vi "PH_DataViewer.Read Data from Disk.vi"(5 "error in":errorcluster) -> (8 "Version":u8, 9 "new file path":path, 10 "Data Vers 1":T31 {"BNC555s"."BNC555 ConfigData"."Configuration"."System"."To Gate Polarity" items=["Low", "High"]; "BNC555s"."BNC555 ConfigData"."Configuration"."System"."To Trigger Edge" items=["Rising", "Falling"]; "BNC555s"."BNC555 ConfigData"."Configuration"."System"."To Trigger Threshold" min=0.2 max=12 step=0.01 format="%.2f"; "BNC555s"."BNC555 ConfigData"."Configuration"."System"."To DCycle Off Count" min=1 max=50000 step=1; "BNC555s"."BNC555 ConfigData"."Configuration"."System"."To DCycle On Count" min=1 max=50000 step=1; "BNC555s"."BNC555 ConfigData"."Configuration"."System"."To Burst Count" min=1 max=50000 step=1; "BNC555s"."BNC555 ConfigData"."Configuration"."System"."To Trigger Mode" items=["Disabled", "Trigger", "Gate"]; "BNC555s"."BNC555 ConfigData"."Configuration"."System"."To Mode" items=["Normal", "Single", "Burst", "DCycle"]; "BNC555s"."BNC555 ConfigData"."Configuration"."System"."To Period" min=1e-06 max=20.0 step=1e-07 format="%.7f"; "BNC555s"."BNC555 ConfigData"."Configuration"."System"."To State" items=["Disabled", "Enable"]; "BNC555s"."BNC555 ConfigData"."Channel Array"."Channel Setup"."Ch Divide By Count" min=1 max=50000 step=1; "BNC555s"."BNC555 ConfigData"."Channel Array"."Channel Setup"."Ch Burst Count" min=1 max=50000 step=1; "BNC555s"."BNC555 ConfigData"."Channel Array"."Channel Setup"."Ch Mode" items=["Normal", "Single", "Burst", "Divide by"]; "BNC555s"."BNC555 ConfigData"."Channel Array"."Channel Setup"."Ch Gate" items=["Disabled", "Enabled"]; "BNC555s"."BNC555 ConfigData"."Channel Array"."Channel Setup"."Ch Gate Polarity" items=["Normal", "Complement"]; "BNC555s"."BNC555 ConfigData"."Channel Array"."Channel Setup"."Ch Polarity" items=["Normal", "Complement"]; "BNC555s"."BNC555 ConfigData"."Channel Array"."Channel Setup"."Ch Amplitude" min=1.99 max=12 step=0.01 format="%.2f"; "BNC555s"."BNC555 ConfigData"."Channel Array"."Channel Setup"."Ch Output" items=["TTL", "Adjustable"]; "BNC555s"."BNC555 ConfigData"."Channel Array"."Channel Setup"."Ch Delay" min=0.0 max=20.0 step=1e-09 format="%.9f"; "BNC555s"."BNC555 ConfigData"."Channel Array"."Channel Setup"."Ch Width" min=4e-09 max=20.0 step=1e-09 format="%.9f"; "BNC555s"."BNC555 ConfigData"."Channel Array"."Channel Setup"."Ch State" items=["Disabled", "Enable"]; "PP PUs"."State" items=["no info", "off/false/out", "on/true/in", "Failure", "Alarm", "Status 1", "Status 2", "Status 3"]; "Chillers"."State Niveau" items=["no info", "off/false", "on/true", "Failure", "Alarm"]; "Chillers"."State Temperature" items=["no info", "off/false", "on/true", "Failure", "Alarm"]; "Chillers"."State Conductivity" items=["no info", "off/false", "on/true", "Failure", "Alarm"]; "Chillers"."State Flow" items=["no info", "off/false", "on/true", "Failure", "Alarm"]; "Mercury Monitors"."Concentration [mg/m³]" format="%#_9g"; "Mercury Monitors"."State Alarm" items=["no info", "off/false", "on/true", "Failure", "Alarm"]; "Mercury Monitors"."State On/Off" items=["no info", "off/false", "on/true", "Failure", "Alarm"]; "Img Operators"."Energy"."State" items=["no info", "off/false", "on/true", "Failure", "Alarm"]; "Img Operators"."Cam Settings"."Serial Number" format="%#_12g"; "Img Operators"."Calibration"."Calibration data - Version 1"."Cam Settings"."Serial Number" format="%#_12g"; "Img Operators"."Calibration"."Status" items=["no info", "off/false", "on/true", "Failure", "Alarm"]; "Cams"."Cam Settings"."Serial Number" format="%#_12g"; "Powermeters"."Device State" items=["no info", "off/false", "on/true", "Failure", "Alarm"]; "Calorimeters"."PH Calorimeter Device Config"."Channel Gain" items=["Range: +/- 10 V", "Range: +/- 2.5 V ", "Range: +/- 1 V", "Range: +/- 0.25 V", "Range: +/- 0.1 V", "Range: +/- 0.025 V"]; "Calorimeters"."PH Calorimeter Device Config"."Channel" items=["Channel 1", "Channel 2", "Channel 3", "Channel 4", "Channel 5", "Channel 6", "Channel 7", "Channel 8", "Channel 9", "Channel 10", "Channel 11", "Channel 12", "Channel 13", "Channel 14", "Channel 15", "Channel 16"]; "Black Boxes"."Status" items=["no info", "off/false", "on/true", "Failure", "Alarm", "Status 1", "Status 2", "Status 3"]}, 12 "Data Vers 2":T32 {"SRDG535s"."Trigger Settings"."Burst Period" min=4 max=32766; "SRDG535s"."Trigger Settings"."Internal/Burst Rate (Hz)" min=0.001 max=1000000.0 format="%.3f"; "SRDG535s"."Trigger Settings"."external level (V)" min=-2.56 max=2.56 format="%.2f"; "SRDG535s"."Trigger Settings"."burst count" min=2 max=32766; "SRDG535s"."Trigger Settings"."trigger" scale=0.0..4.0; "SRDG535s"."Output Settings"."CH CD"."Mode" items=["TTL", "NIM", "ECL", "VAR"]; "SRDG535s"."Output Settings"."CH CD"."Offset (V)" min=-3.0 max=4.0 format="%.2f"; "SRDG535s"."Output Settings"."CH CD"."Amplitude (V)" min=-3.0 max=4.0 format="%.2f"; "SRDG535s"."Output Settings"."CH D"."Mode" items=["TTL", "NIM", "ECL", "VAR"]; "SRDG535s"."Output Settings"."CH D"."Offset (V)" min=-3.0 max=4.0 format="%.2f"; "SRDG535s"."Output Settings"."CH D"."Amplitude (V)" min=-3.0 max=4.0 format="%.2f"; "SRDG535s"."Output Settings"."CH C"."Mode" items=["TTL", "NIM", "ECL", "VAR"]; "SRDG535s"."Output Settings"."CH C"."Offset (V)" min=-3.0 max=4.0 format="%.2f"; "SRDG535s"."Output Settings"."CH C"."Amplitude (V)" min=-3.0 max=4.0 format="%.2f"; "SRDG535s"."Output Settings"."CH AB"."Mode" items=["TTL", "NIM", "ECL", "VAR"]; "SRDG535s"."Output Settings"."CH AB"."Offset (V)" min=-3.0 max=4.0 format="%.2f"; "SRDG535s"."Output Settings"."CH AB"."Amplitude (V)" min=-3.0 max=4.0 format="%.2f"; "SRDG535s"."Output Settings"."CH B"."Mode" items=["TTL", "NIM", "ECL", "VAR"]; "SRDG535s"."Output Settings"."CH B"."Offset (V)" min=-3.0 max=4.0 format="%.2f"; "SRDG535s"."Output Settings"."CH B"."Amplitude (V)" min=-3.0 max=4.0 format="%.2f"; "SRDG535s"."Output Settings"."CH A"."Mode" items=["TTL", "NIM", "ECL", "VAR"]; "SRDG535s"."Output Settings"."CH A"."Offset (V)" min=-3.0 max=4.0 format="%.2f"; "SRDG535s"."Output Settings"."CH A"."Amplitude (V)" min=-3.0 max=4.0 format="%.2f"; "SRDG535s"."Output Settings"."CH T0"."Mode" items=["TTL", "NIM", "ECL", "VAR"]; "SRDG535s"."Output Settings"."CH T0"."Offset (V)" min=-3.0 max=4.0 format="%.2f"; "SRDG535s"."Output Settings"."CH T0"."Amplitude (V)" min=-3.0 max=4.0 format="%.2f"; "SRDG535s"."Delay Settings"."CH D"."Delay (s)" format="%#_13g"; "SRDG535s"."Delay Settings"."CH D"."rel to" scale=0.0..3.0; "SRDG535s"."Delay Settings"."CH C"."Delay (s)" format="%#_13g"; "SRDG535s"."Delay Settings"."CH C"."rel to" scale=0.0..3.0; "SRDG535s"."Delay Settings"."CH B"."Delay (s)" format="%#_13g"; "SRDG535s"."Delay Settings"."CH B"."rel to" scale=0.0..3.0; "SRDG535s"."Delay Settings"."CH A"."Delay (s)" format="%#_13g"; "SRDG535s"."Delay Settings"."CH A"."rel to" scale=0.0..3.0; "BNC555s"."BNC555 ConfigData"."Configuration"."System"."To Gate Polarity" items=["Low", "High"]; "BNC555s"."BNC555 ConfigData"."Configuration"."System"."To Trigger Edge" items=["Rising", "Falling"]; "BNC555s"."BNC555 ConfigData"."Configuration"."System"."To Trigger Threshold" min=0.2 max=12 step=0.01 format="%.2f"; "BNC555s"."BNC555 ConfigData"."Configuration"."System"."To DCycle Off Count" min=1 max=50000 step=1; "BNC555s"."BNC555 ConfigData"."Configuration"."System"."To DCycle On Count" min=1 max=50000 step=1; "BNC555s"."BNC555 ConfigData"."Configuration"."System"."To Burst Count" min=1 max=50000 step=1; "BNC555s"."BNC555 ConfigData"."Configuration"."System"."To Trigger Mode" items=["Disabled", "Trigger", "Gate"]; "BNC555s"."BNC555 ConfigData"."Configuration"."System"."To Mode" items=["Normal", "Single", "Burst", "DCycle"]; "BNC555s"."BNC555 ConfigData"."Configuration"."System"."To Period" min=1e-06 max=20.0 step=1e-07 format="%.7f"; "BNC555s"."BNC555 ConfigData"."Configuration"."System"."To State" items=["Disabled", "Enable"]; "BNC555s"."BNC555 ConfigData"."Channel Array"."Channel Setup"."Ch Divide By Count" min=1 max=50000 step=1; "BNC555s"."BNC555 ConfigData"."Channel Array"."Channel Setup"."Ch Burst Count" min=1 max=50000 step=1; "BNC555s"."BNC555 ConfigData"."Channel Array"."Channel Setup"."Ch Mode" items=["Normal", "Single", "Burst", "Divide by"]; "BNC555s"."BNC555 ConfigData"."Channel Array"."Channel Setup"."Ch Gate" items=["Disabled", "Enabled"]; "BNC555s"."BNC555 ConfigData"."Channel Array"."Channel Setup"."Ch Gate Polarity" items=["Normal", "Complement"]; "BNC555s"."BNC555 ConfigData"."Channel Array"."Channel Setup"."Ch Polarity" items=["Normal", "Complement"]; "BNC555s"."BNC555 ConfigData"."Channel Array"."Channel Setup"."Ch Amplitude" min=1.99 max=12 step=0.01 format="%.2f"; "BNC555s"."BNC555 ConfigData"."Channel Array"."Channel Setup"."Ch Output" items=["TTL", "Adjustable"]; "BNC555s"."BNC555 ConfigData"."Channel Array"."Channel Setup"."Ch Delay" min=0.0 max=20.0 step=1e-09 format="%.9f"; "BNC555s"."BNC555 ConfigData"."Channel Array"."Channel Setup"."Ch Width" min=4e-09 max=20.0 step=1e-09 format="%.9f"; "BNC555s"."BNC555 ConfigData"."Channel Array"."Channel Setup"."Ch State" items=["Disabled", "Enable"]; "PP PUs"."State" items=["no info", "off/false/out", "on/true/in", "Failure", "Alarm", "Status 1", "Status 2", "Status 3"]; "Chillers"."State Niveau" items=["no info", "off/false", "on/true", "Failure", "Alarm"]; "Chillers"."State Temperature" items=["no info", "off/false", "on/true", "Failure", "Alarm"]; "Chillers"."State Conductivity" items=["no info", "off/false", "on/true", "Failure", "Alarm"]; "Chillers"."State Flow" items=["no info", "off/false", "on/true", "Failure", "Alarm"]; "Mercury Monitors"."Concentration [mg/m³]" format="%#_9g"; "Mercury Monitors"."State Alarm" items=["no info", "off/false", "on/true", "Failure", "Alarm"]; "Mercury Monitors"."State On/Off" items=["no info", "off/false", "on/true", "Failure", "Alarm"]; "Img Operators"."Energy"."State" items=["no info", "off/false", "on/true", "Failure", "Alarm"]; "Img Operators"."Cam Settings"."Serial Number" format="%#_12g"; "Img Operators"."Calibration"."Calibration data - Version 1"."Cam Settings"."Serial Number" format="%#_12g"; "Img Operators"."Calibration"."Status" items=["no info", "off/false", "on/true", "Failure", "Alarm"]; "Cams"."Cam Settings"."Serial Number" format="%#_12g"; "Powermeters"."Device State" items=["no info", "off/false", "on/true", "Failure", "Alarm"]; "Calorimeters"."PH Calorimeter Device Config"."Channel Gain" items=["Range: +/- 10 V", "Range: +/- 2.5 V ", "Range: +/- 1 V", "Range: +/- 0.25 V", "Range: +/- 0.1 V", "Range: +/- 0.025 V"]; "Calorimeters"."PH Calorimeter Device Config"."Channel" items=["Channel 1", "Channel 2", "Channel 3", "Channel 4", "Channel 5", "Channel 6", "Channel 7", "Channel 8", "Channel 9", "Channel 10", "Channel 11", "Channel 12", "Channel 13", "Channel 14", "Channel 15", "Channel 16"]; "Black Boxes"."Status" items=["no info", "off/false", "on/true", "Failure", "Alarm", "Status 1", "Status 2", "Status 3"]}, 14 "Data Vers 3":T33 {"Backreflection Meas"."Waveform Data"."Initial X" format="%.2e"; "SRDG535s"."Trigger Settings"."Burst Period" min=4 max=32766; "SRDG535s"."Trigger Settings"."Internal/Burst Rate (Hz)" min=0.001 max=1000000.0 format="%.3f"; "SRDG535s"."Trigger Settings"."external level (V)" min=-2.56 max=2.56 format="%.2f"; "SRDG535s"."Trigger Settings"."burst count" min=2 max=32766; "SRDG535s"."Trigger Settings"."trigger" scale=0.0..4.0; "SRDG535s"."Output Settings"."CH CD"."Mode" items=["TTL", "NIM", "ECL", "VAR"]; "SRDG535s"."Output Settings"."CH CD"."Offset (V)" min=-3.0 max=4.0 format="%.2f"; "SRDG535s"."Output Settings"."CH CD"."Amplitude (V)" min=-3.0 max=4.0 format="%.2f"; "SRDG535s"."Output Settings"."CH D"."Mode" items=["TTL", "NIM", "ECL", "VAR"]; "SRDG535s"."Output Settings"."CH D"."Offset (V)" min=-3.0 max=4.0 format="%.2f"; "SRDG535s"."Output Settings"."CH D"."Amplitude (V)" min=-3.0 max=4.0 format="%.2f"; "SRDG535s"."Output Settings"."CH C"."Mode" items=["TTL", "NIM", "ECL", "VAR"]; "SRDG535s"."Output Settings"."CH C"."Offset (V)" min=-3.0 max=4.0 format="%.2f"; "SRDG535s"."Output Settings"."CH C"."Amplitude (V)" min=-3.0 max=4.0 format="%.2f"; "SRDG535s"."Output Settings"."CH AB"."Mode" items=["TTL", "NIM", "ECL", "VAR"]; "SRDG535s"."Output Settings"."CH AB"."Offset (V)" min=-3.0 max=4.0 format="%.2f"; "SRDG535s"."Output Settings"."CH AB"."Amplitude (V)" min=-3.0 max=4.0 format="%.2f"; "SRDG535s"."Output Settings"."CH B"."Mode" items=["TTL", "NIM", "ECL", "VAR"]; "SRDG535s"."Output Settings"."CH B"."Offset (V)" min=-3.0 max=4.0 format="%.2f"; "SRDG535s"."Output Settings"."CH B"."Amplitude (V)" min=-3.0 max=4.0 format="%.2f"; "SRDG535s"."Output Settings"."CH A"."Mode" items=["TTL", "NIM", "ECL", "VAR"]; "SRDG535s"."Output Settings"."CH A"."Offset (V)" min=-3.0 max=4.0 format="%.2f"; "SRDG535s"."Output Settings"."CH A"."Amplitude (V)" min=-3.0 max=4.0 format="%.2f"; "SRDG535s"."Output Settings"."CH T0"."Mode" items=["TTL", "NIM", "ECL", "VAR"]; "SRDG535s"."Output Settings"."CH T0"."Offset (V)" min=-3.0 max=4.0 format="%.2f"; "SRDG535s"."Output Settings"."CH T0"."Amplitude (V)" min=-3.0 max=4.0 format="%.2f"; "SRDG535s"."Delay Settings"."CH D"."Delay (s)" format="%#_13g"; "SRDG535s"."Delay Settings"."CH D"."rel to" scale=0.0..3.0; "SRDG535s"."Delay Settings"."CH C"."Delay (s)" format="%#_13g"; "SRDG535s"."Delay Settings"."CH C"."rel to" scale=0.0..3.0; "SRDG535s"."Delay Settings"."CH B"."Delay (s)" format="%#_13g"; "SRDG535s"."Delay Settings"."CH B"."rel to" scale=0.0..3.0; "SRDG535s"."Delay Settings"."CH A"."Delay (s)" format="%#_13g"; "SRDG535s"."Delay Settings"."CH A"."rel to" scale=0.0..3.0; "BNC555s"."BNC555 ConfigData"."Configuration"."System"."To Gate Polarity" items=["Low", "High"]; "BNC555s"."BNC555 ConfigData"."Configuration"."System"."To Trigger Edge" items=["Rising", "Falling"]; "BNC555s"."BNC555 ConfigData"."Configuration"."System"."To Trigger Threshold" min=0.2 max=12 step=0.01 format="%.2f"; "BNC555s"."BNC555 ConfigData"."Configuration"."System"."To DCycle Off Count" min=1 max=50000 step=1; "BNC555s"."BNC555 ConfigData"."Configuration"."System"."To DCycle On Count" min=1 max=50000 step=1; "BNC555s"."BNC555 ConfigData"."Configuration"."System"."To Burst Count" min=1 max=50000 step=1; "BNC555s"."BNC555 ConfigData"."Configuration"."System"."To Trigger Mode" items=["Disabled", "Trigger", "Gate"]; "BNC555s"."BNC555 ConfigData"."Configuration"."System"."To Mode" items=["Normal", "Single", "Burst", "DCycle"]; "BNC555s"."BNC555 ConfigData"."Configuration"."System"."To Period" min=1e-06 max=20.0 step=1e-07 format="%.7f"; "BNC555s"."BNC555 ConfigData"."Configuration"."System"."To State" items=["Disabled", "Enable"]; "BNC555s"."BNC555 ConfigData"."Channel Array"."Channel Setup"."Ch Divide By Count" min=1 max=50000 step=1; "BNC555s"."BNC555 ConfigData"."Channel Array"."Channel Setup"."Ch Burst Count" min=1 max=50000 step=1; "BNC555s"."BNC555 ConfigData"."Channel Array"."Channel Setup"."Ch Mode" items=["Normal", "Single", "Burst", "Divide by"]; "BNC555s"."BNC555 ConfigData"."Channel Array"."Channel Setup"."Ch Gate" items=["Disabled", "Enabled"]; "BNC555s"."BNC555 ConfigData"."Channel Array"."Channel Setup"."Ch Gate Polarity" items=["Normal", "Complement"]; "BNC555s"."BNC555 ConfigData"."Channel Array"."Channel Setup"."Ch Polarity" items=["Normal", "Complement"]; "BNC555s"."BNC555 ConfigData"."Channel Array"."Channel Setup"."Ch Amplitude" min=1.99 max=12 step=0.01 format="%.2f"; "BNC555s"."BNC555 ConfigData"."Channel Array"."Channel Setup"."Ch Output" items=["TTL", "Adjustable"]; "BNC555s"."BNC555 ConfigData"."Channel Array"."Channel Setup"."Ch Delay" min=0.0 max=20.0 step=1e-09 format="%.9f"; "BNC555s"."BNC555 ConfigData"."Channel Array"."Channel Setup"."Ch Width" min=4e-09 max=20.0 step=1e-09 format="%.9f"; "BNC555s"."BNC555 ConfigData"."Channel Array"."Channel Setup"."Ch State" items=["Disabled", "Enable"]; "PP PUs"."State" items=["no info", "off/false/out", "on/true/in", "Failure", "Alarm", "Status 1", "Status 2", "Status 3"]; "Chillers"."State Niveau" items=["no info", "off/false", "on/true", "Failure", "Alarm"]; "Chillers"."State Temperature" items=["no info", "off/false", "on/true", "Failure", "Alarm"]; "Chillers"."State Conductivity" items=["no info", "off/false", "on/true", "Failure", "Alarm"]; "Chillers"."State Flow" items=["no info", "off/false", "on/true", "Failure", "Alarm"]; "Mercury Monitors"."Concentration [mg/m³]" format="%#_9g"; "Mercury Monitors"."State Alarm" items=["no info", "off/false", "on/true", "Failure", "Alarm"]; "Mercury Monitors"."State On/Off" items=["no info", "off/false", "on/true", "Failure", "Alarm"]; "Img Operators"."Energy"."State" items=["no info", "off/false", "on/true", "Failure", "Alarm"]; "Img Operators"."Cam Settings"."Serial Number" format="%#_12g"; "Img Operators"."Calibration"."Calibration data - Version 1"."Cam Settings"."Serial Number" format="%#_12g"; "Img Operators"."Calibration"."Status" items=["no info", "off/false", "on/true", "Failure", "Alarm"]; "Cams"."Cam Settings"."Serial Number" format="%#_12g"; "Powermeters"."Device State" items=["no info", "off/false", "on/true", "Failure", "Alarm"]; "Calorimeters"."PH Calorimeter Device Config"."Channel Gain" items=["Range: +/- 10 V", "Range: +/- 2.5 V ", "Range: +/- 1 V", "Range: +/- 0.25 V", "Range: +/- 0.1 V", "Range: +/- 0.025 V"]; "Calorimeters"."PH Calorimeter Device Config"."Channel" items=["Channel 1", "Channel 2", "Channel 3", "Channel 4", "Channel 5", "Channel 6", "Channel 7", "Channel 8", "Channel 9", "Channel 10", "Channel 11", "Channel 12", "Channel 13", "Channel 14", "Channel 15", "Channel 16"]; "Black Boxes"."Status" items=["no info", "off/false", "on/true", "Failure", "Alarm", "Status 1", "Status 2", "Status 3"]}, 15 "Data Vers 4":T1={"Black Boxes"=[], "Calorimeters"=[], "Current Meas'"=[], "Powermeters"=[], "Cams"=[], "Img Operators"=[], "Mercury Monitors"=[], "Chillers"=[], "Triggers"=[], "Vac Controls"=[], "PP PUs"=[], "BNC555s"=[], "SRDG535s"=[], "Sequencer Data"={"Instance"="", "Snapshot: Date"="N/A", "Snapshot: Time"="N/A", "Shot Comment"=""}, "Backreflection Meas"=[], "OO Spectrometer"=[]} {"Backreflection Meas"."Waveform Data"."Initial X" format="%.2e"; "SRDG535s"."Trigger Settings"."Burst Period" min=4 max=32766; "SRDG535s"."Trigger Settings"."Internal/Burst Rate (Hz)" min=0.001 max=1000000.0 format="%.3f"; "SRDG535s"."Trigger Settings"."external level (V)" min=-2.56 max=2.56 format="%.2f"; "SRDG535s"."Trigger Settings"."burst count" min=2 max=32766; "SRDG535s"."Trigger Settings"."trigger" scale=0.0..4.0; "SRDG535s"."Output Settings"."CH CD"."Mode" items=["TTL", "NIM", "ECL", "VAR"]; "SRDG535s"."Output Settings"."CH CD"."Offset (V)" min=-3.0 max=4.0 format="%.2f"; "SRDG535s"."Output Settings"."CH CD"."Amplitude (V)" min=-3.0 max=4.0 format="%.2f"; "SRDG535s"."Output Settings"."CH D"."Mode" items=["TTL", "NIM", "ECL", "VAR"]; "SRDG535s"."Output Settings"."CH D"."Offset (V)" min=-3.0 max=4.0 format="%.2f"; "SRDG535s"."Output Settings"."CH D"."Amplitude (V)" min=-3.0 max=4.0 format="%.2f"; "SRDG535s"."Output Settings"."CH C"."Mode" items=["TTL", "NIM", "ECL", "VAR"]; "SRDG535s"."Output Settings"."CH C"."Offset (V)" min=-3.0 max=4.0 format="%.2f"; "SRDG535s"."Output Settings"."CH C"."Amplitude (V)" min=-3.0 max=4.0 format="%.2f"; "SRDG535s"."Output Settings"."CH AB"."Mode" items=["TTL", "NIM", "ECL", "VAR"]; "SRDG535s"."Output Settings"."CH AB"."Offset (V)" min=-3.0 max=4.0 format="%.2f"; "SRDG535s"."Output Settings"."CH AB"."Amplitude (V)" min=-3.0 max=4.0 format="%.2f"; "SRDG535s"."Output Settings"."CH B"."Mode" items=["TTL", "NIM", "ECL", "VAR"]; "SRDG535s"."Output Settings"."CH B"."Offset (V)" min=-3.0 max=4.0 format="%.2f"; "SRDG535s"."Output Settings"."CH B"."Amplitude (V)" min=-3.0 max=4.0 format="%.2f"; "SRDG535s"."Output Settings"."CH A"."Mode" items=["TTL", "NIM", "ECL", "VAR"]; "SRDG535s"."Output Settings"."CH A"."Offset (V)" min=-3.0 max=4.0 format="%.2f"; "SRDG535s"."Output Settings"."CH A"."Amplitude (V)" min=-3.0 max=4.0 format="%.2f"; "SRDG535s"."Output Settings"."CH T0"."Mode" items=["TTL", "NIM", "ECL", "VAR"]; "SRDG535s"."Output Settings"."CH T0"."Offset (V)" min=-3.0 max=4.0 format="%.2f"; "SRDG535s"."Output Settings"."CH T0"."Amplitude (V)" min=-3.0 max=4.0 format="%.2f"; "SRDG535s"."Delay Settings"."CH D"."Delay (s)" format="%#_13g"; "SRDG535s"."Delay Settings"."CH D"."rel to" scale=0.0..3.0; "SRDG535s"."Delay Settings"."CH C"."Delay (s)" format="%#_13g"; "SRDG535s"."Delay Settings"."CH C"."rel to" scale=0.0..3.0; "SRDG535s"."Delay Settings"."CH B"."Delay (s)" format="%#_13g"; "SRDG535s"."Delay Settings"."CH B"."rel to" scale=0.0..3.0; "SRDG535s"."Delay Settings"."CH A"."Delay (s)" format="%#_13g"; "SRDG535s"."Delay Settings"."CH A"."rel to" scale=0.0..3.0; "BNC555s"."BNC555 ConfigData"."Configuration"."System"."To Gate Polarity" items=["Low", "High"]; "BNC555s"."BNC555 ConfigData"."Configuration"."System"."To Trigger Edge" items=["Rising", "Falling"]; "BNC555s"."BNC555 ConfigData"."Configuration"."System"."To Trigger Threshold" min=0.2 max=12 step=0.01 format="%.2f"; "BNC555s"."BNC555 ConfigData"."Configuration"."System"."To DCycle Off Count" min=1 max=50000 step=1; "BNC555s"."BNC555 ConfigData"."Configuration"."System"."To DCycle On Count" min=1 max=50000 step=1; "BNC555s"."BNC555 ConfigData"."Configuration"."System"."To Burst Count" min=1 max=50000 step=1; "BNC555s"."BNC555 ConfigData"."Configuration"."System"."To Trigger Mode" items=["Disabled", "Trigger", "Gate"]; "BNC555s"."BNC555 ConfigData"."Configuration"."System"."To Mode" items=["Normal", "Single", "Burst", "DCycle"]; "BNC555s"."BNC555 ConfigData"."Configuration"."System"."To Period" min=1e-06 max=20.0 step=1e-07 format="%.7f"; "BNC555s"."BNC555 ConfigData"."Configuration"."System"."To State" items=["Disabled", "Enable"]; "BNC555s"."BNC555 ConfigData"."Channel Array"."Channel Setup"."Ch Divide By Count" min=1 max=50000 step=1; "BNC555s"."BNC555 ConfigData"."Channel Array"."Channel Setup"."Ch Burst Count" min=1 max=50000 step=1; "BNC555s"."BNC555 ConfigData"."Channel Array"."Channel Setup"."Ch Mode" items=["Normal", "Single", "Burst", "Divide by"]; "BNC555s"."BNC555 ConfigData"."Channel Array"."Channel Setup"."Ch Gate" items=["Disabled", "Enabled"]; "BNC555s"."BNC555 ConfigData"."Channel Array"."Channel Setup"."Ch Gate Polarity" items=["Normal", "Complement"]; "BNC555s"."BNC555 ConfigData"."Channel Array"."Channel Setup"."Ch Polarity" items=["Normal", "Complement"]; "BNC555s"."BNC555 ConfigData"."Channel Array"."Channel Setup"."Ch Amplitude" min=1.99 max=12 step=0.01 format="%.2f"; "BNC555s"."BNC555 ConfigData"."Channel Array"."Channel Setup"."Ch Output" items=["TTL", "Adjustable"]; "BNC555s"."BNC555 ConfigData"."Channel Array"."Channel Setup"."Ch Delay" min=0.0 max=20.0 step=1e-09 format="%.9f"; "BNC555s"."BNC555 ConfigData"."Channel Array"."Channel Setup"."Ch Width" min=4e-09 max=20.0 step=1e-09 format="%.9f"; "BNC555s"."BNC555 ConfigData"."Channel Array"."Channel Setup"."Ch State" items=["Disabled", "Enable"]; "PP PUs"."State" items=["no info", "off/false/out", "on/true/in", "Failure", "Alarm", "Status 1", "Status 2", "Status 3"]; "Chillers"."State Niveau" items=["no info", "off/false", "on/true", "Failure", "Alarm"]; "Chillers"."State Temperature" items=["no info", "off/false", "on/true", "Failure", "Alarm"]; "Chillers"."State Conductivity" items=["no info", "off/false", "on/true", "Failure", "Alarm"]; "Chillers"."State Flow" items=["no info", "off/false", "on/true", "Failure", "Alarm"]; "Mercury Monitors"."Concentration [mg/m³]" format="%#_9g"; "Mercury Monitors"."State Alarm" items=["no info", "off/false", "on/true", "Failure", "Alarm"]; "Mercury Monitors"."State On/Off" items=["no info", "off/false", "on/true", "Failure", "Alarm"]; "Img Operators"."Energy"."State" items=["no info", "off/false", "on/true", "Failure", "Alarm"]; "Img Operators"."Cam Settings"."Serial Number" format="%#_12g"; "Img Operators"."Calibration"."Calibration data - Version 1"."Cam Settings"."Serial Number" format="%#_12g"; "Img Operators"."Calibration"."Status" items=["no info", "off/false", "on/true", "Failure", "Alarm"]; "Cams"."Cam Settings"."Serial Number" format="%#_12g"; "Powermeters"."Device State" items=["no info", "off/false", "on/true", "Failure", "Alarm"]; "Calorimeters"."PH Calorimeter Device Config"."Channel Gain" items=["Range: +/- 10 V", "Range: +/- 2.5 V ", "Range: +/- 1 V", "Range: +/- 0.25 V", "Range: +/- 0.1 V", "Range: +/- 0.025 V"]; "Calorimeters"."PH Calorimeter Device Config"."Channel" items=["Channel 1", "Channel 2", "Channel 3", "Channel 4", "Channel 5", "Channel 6", "Channel 7", "Channel 8", "Channel 9", "Channel 10", "Channel 11", "Channel 12", "Channel 13", "Channel 14", "Channel 15", "Channel 16"]; "Black Boxes"."Status" items=["no info", "off/false", "on/true", "Failure", "Alarm", "Status 1", "Status 2", "Status 3"]}, 19 "error IO":errorcluster)   [LabVIEW 2014, in "PH_DataViewer.lvlib"]
doc: "This is the VI which reads the data from hard disk. It handles different versions of data cluster."
uses:
  PH_DataViewer.lvlib
  PH_Blackbox.Data.ctl
  PH_Calorimater_USB.Data.ctl
  PH_Calorimeter_USB/PH_Calorimeter_USB.Device Config.ctl
  PH_Calorimeter_USB/PH_Calorimeter_USB.Channel.ctl
  PH_Calorimeter_USB/PH_Calorimeter_USB.Channel Gain.ctl
  PH_CurrentMeas.Data.ctl
  PH_gentec_Powermeter.Data.ctl
  PH_DataViewer.Device State.ctl
  PH_IEEE1394Camera.Data.ctl
  PH_IEEE1394Camera.Settings.ctl
  PH_ImageOperator.Data.ctl
  PH_Vision/PH_ImageCalibrator/PH_ImageCalibrator.Calibration Data - Version 1.ctl
  PH_Vision/PH_ImageOperator/PH_ImageOperator.Beam Analysis Data.ctl
  PH_Mercury_Monitor.Data.ctl
  PH_PA_Chiller.Data.ctl
  PH_PP_Trigger.Data.ctl
  PH_VacuumControl.Data.ctl
  PH_Common.PP PU Data.ctl
  PH_Basics/PH_StatusHandler/PH_StatusHandler.Status.ctl
  BNC555.Data.ctl
  PHELIX_Data_Vers2.ctl
  PH_Common.PP PU Data Vers2.ctl
  SRDG535.Data.ctl
  CS_DigitalIO/SRDG535/SRDG535.Delay.ctl
  CS_DigitalIO/SRDG535/SRDG535.Output.ctl
  CS_DigitalIO/SRDG535/SRDG535.Channel Output.ctl
  CS_DigitalIO/SRDG535/SRDG535.Trigger.ctl
  PH_Sequencer.Data.ctl
  PHELIX_Data_Vers3.ctl
  PH_BackreflectionMeas.Data.ctl
  PHELIX_Data_Vers4.ctl
  PH_OceanOpticsSpectrometer.Data.ctl
  PH_Calorimeter_USB/PH_Calorimeter_USB.lvlib
  PH_Vision/PH_ImageOperator/PH_ImageOperator.lvlib
  PH_Basics/PH_StatusHandler/PH_StatusHandler.lvlib
  CS_DigitalIO/SRDG535/SRDG535.lvlib
  PH_Vision/PH_ImageCalibrator/PH_ImageCalibrator.lvlib
panel:
  in  "Version 4":T1={"Black Boxes"=[], "Calorimeters"=[], "Current Meas'"=[], "Powermeters"=[], "Cams"=[], "Img Operators"=[], "Mercury Monitors"=[], "Chillers"=[], "Triggers"=[], "Vac Controls"=[], "PP PUs"=[], "BNC555s"=[], "SRDG535s"=[], "Sequencer Data"={"Instance"="", "Snapshot: Date"="N/A", "Snapshot: Time"="N/A", "Shot Comment"=""}, "Backreflection Meas"=[], "OO Spectrometer"=[]} {"Backreflection Meas"."Waveform Data"."Initial X" format="%.2e"; "SRDG535s"."Trigger Settings"."Burst Period" min=4 max=32766; "SRDG535s"."Trigger Settings"."Internal/Burst Rate (Hz)" min=0.001 max=1000000.0 format="%.3f"; "SRDG535s"."Trigger Settings"."external level (V)" min=-2.56 max=2.56 format="%.2f"; "SRDG535s"."Trigger Settings"."burst count" min=2 max=32766; "SRDG535s"."Trigger Settings"."trigger" scale=0.0..4.0; "SRDG535s"."Output Settings"."CH CD"."Mode" items=["TTL", "NIM", "ECL", "VAR"]; "SRDG535s"."Output Settings"."CH CD"."Offset (V)" min=-3.0 max=4.0 format="%.2f"; "SRDG535s"."Output Settings"."CH CD"."Amplitude (V)" min=-3.0 max=4.0 format="%.2f"; "SRDG535s"."Output Settings"."CH D"."Mode" items=["TTL", "NIM", "ECL", "VAR"]; "SRDG535s"."Output Settings"."CH D"."Offset (V)" min=-3.0 max=4.0 format="%.2f"; "SRDG535s"."Output Settings"."CH D"."Amplitude (V)" min=-3.0 max=4.0 format="%.2f"; "SRDG535s"."Output Settings"."CH C"."Mode" items=["TTL", "NIM", "ECL", "VAR"]; "SRDG535s"."Output Settings"."CH C"."Offset (V)" min=-3.0 max=4.0 format="%.2f"; "SRDG535s"."Output Settings"."CH C"."Amplitude (V)" min=-3.0 max=4.0 format="%.2f"; "SRDG535s"."Output Settings"."CH AB"."Mode" items=["TTL", "NIM", "ECL", "VAR"]; "SRDG535s"."Output Settings"."CH AB"."Offset (V)" min=-3.0 max=4.0 format="%.2f"; "SRDG535s"."Output Settings"."CH AB"."Amplitude (V)" min=-3.0 max=4.0 format="%.2f"; "SRDG535s"."Output Settings"."CH B"."Mode" items=["TTL", "NIM", "ECL", "VAR"]; "SRDG535s"."Output Settings"."CH B"."Offset (V)" min=-3.0 max=4.0 format="%.2f"; "SRDG535s"."Output Settings"."CH B"."Amplitude (V)" min=-3.0 max=4.0 format="%.2f"; "SRDG535s"."Output Settings"."CH A"."Mode" items=["TTL", "NIM", "ECL", "VAR"]; "SRDG535s"."Output Settings"."CH A"."Offset (V)" min=-3.0 max=4.0 format="%.2f"; "SRDG535s"."Output Settings"."CH A"."Amplitude (V)" min=-3.0 max=4.0 format="%.2f"; "SRDG535s"."Output Settings"."CH T0"."Mode" items=["TTL", "NIM", "ECL", "VAR"]; "SRDG535s"."Output Settings"."CH T0"."Offset (V)" min=-3.0 max=4.0 format="%.2f"; "SRDG535s"."Output Settings"."CH T0"."Amplitude (V)" min=-3.0 max=4.0 format="%.2f"; "SRDG535s"."Delay Settings"."CH D"."Delay (s)" format="%#_13g"; "SRDG535s"."Delay Settings"."CH D"."rel to" scale=0.0..3.0; "SRDG535s"."Delay Settings"."CH C"."Delay (s)" format="%#_13g"; "SRDG535s"."Delay Settings"."CH C"."rel to" scale=0.0..3.0; "SRDG535s"."Delay Settings"."CH B"."Delay (s)" format="%#_13g"; "SRDG535s"."Delay Settings"."CH B"."rel to" scale=0.0..3.0; "SRDG535s"."Delay Settings"."CH A"."Delay (s)" format="%#_13g"; "SRDG535s"."Delay Settings"."CH A"."rel to" scale=0.0..3.0; "BNC555s"."BNC555 ConfigData"."Configuration"."System"."To Gate Polarity" items=["Low", "High"]; "BNC555s"."BNC555 ConfigData"."Configuration"."System"."To Trigger Edge" items=["Rising", "Falling"]; "BNC555s"."BNC555 ConfigData"."Configuration"."System"."To Trigger Threshold" min=0.2 max=12 step=0.01 format="%.2f"; "BNC555s"."BNC555 ConfigData"."Configuration"."System"."To DCycle Off Count" min=1 max=50000 step=1; "BNC555s"."BNC555 ConfigData"."Configuration"."System"."To DCycle On Count" min=1 max=50000 step=1; "BNC555s"."BNC555 ConfigData"."Configuration"."System"."To Burst Count" min=1 max=50000 step=1; "BNC555s"."BNC555 ConfigData"."Configuration"."System"."To Trigger Mode" items=["Disabled", "Trigger", "Gate"]; "BNC555s"."BNC555 ConfigData"."Configuration"."System"."To Mode" items=["Normal", "Single", "Burst", "DCycle"]; "BNC555s"."BNC555 ConfigData"."Configuration"."System"."To Period" min=1e-06 max=20.0 step=1e-07 format="%.7f"; "BNC555s"."BNC555 ConfigData"."Configuration"."System"."To State" items=["Disabled", "Enable"]; "BNC555s"."BNC555 ConfigData"."Channel Array"."Channel Setup"."Ch Divide By Count" min=1 max=50000 step=1; "BNC555s"."BNC555 ConfigData"."Channel Array"."Channel Setup"."Ch Burst Count" min=1 max=50000 step=1; "BNC555s"."BNC555 ConfigData"."Channel Array"."Channel Setup"."Ch Mode" items=["Normal", "Single", "Burst", "Divide by"]; "BNC555s"."BNC555 ConfigData"."Channel Array"."Channel Setup"."Ch Gate" items=["Disabled", "Enabled"]; "BNC555s"."BNC555 ConfigData"."Channel Array"."Channel Setup"."Ch Gate Polarity" items=["Normal", "Complement"]; "BNC555s"."BNC555 ConfigData"."Channel Array"."Channel Setup"."Ch Polarity" items=["Normal", "Complement"]; "BNC555s"."BNC555 ConfigData"."Channel Array"."Channel Setup"."Ch Amplitude" min=1.99 max=12 step=0.01 format="%.2f"; "BNC555s"."BNC555 ConfigData"."Channel Array"."Channel Setup"."Ch Output" items=["TTL", "Adjustable"]; "BNC555s"."BNC555 ConfigData"."Channel Array"."Channel Setup"."Ch Delay" min=0.0 max=20.0 step=1e-09 format="%.9f"; "BNC555s"."BNC555 ConfigData"."Channel Array"."Channel Setup"."Ch Width" min=4e-09 max=20.0 step=1e-09 format="%.9f"; "BNC555s"."BNC555 ConfigData"."Channel Array"."Channel Setup"."Ch State" items=["Disabled", "Enable"]; "PP PUs"."State" items=["no info", "off/false/out", "on/true/in", "Failure", "Alarm", "Status 1", "Status 2", "Status 3"]; "Chillers"."State Niveau" items=["no info", "off/false", "on/true", "Failure", "Alarm"]; "Chillers"."State Temperature" items=["no info", "off/false", "on/true", "Failure", "Alarm"]; "Chillers"."State Conductivity" items=["no info", "off/false", "on/true", "Failure", "Alarm"]; "Chillers"."State Flow" items=["no info", "off/false", "on/true", "Failure", "Alarm"]; "Mercury Monitors"."Concentration [mg/m³]" format="%#_9g"; "Mercury Monitors"."State Alarm" items=["no info", "off/false", "on/true", "Failure", "Alarm"]; "Mercury Monitors"."State On/Off" items=["no info", "off/false", "on/true", "Failure", "Alarm"]; "Img Operators"."Energy"."State" items=["no info", "off/false", "on/true", "Failure", "Alarm"]; "Img Operators"."Cam Settings"."Serial Number" format="%#_12g"; "Img Operators"."Calibration"."Calibration data - Version 1"."Cam Settings"."Serial Number" format="%#_12g"; "Img Operators"."Calibration"."Status" items=["no info", "off/false", "on/true", "Failure", "Alarm"]; "Cams"."Cam Settings"."Serial Number" format="%#_12g"; "Powermeters"."Device State" items=["no info", "off/false", "on/true", "Failure", "Alarm"]; "Calorimeters"."PH Calorimeter Device Config"."Channel Gain" items=["Range: +/- 10 V", "Range: +/- 2.5 V ", "Range: +/- 1 V", "Range: +/- 0.25 V", "Range: +/- 0.1 V", "Range: +/- 0.025 V"]; "Calorimeters"."PH Calorimeter Device Config"."Channel" items=["Channel 1", "Channel 2", "Channel 3", "Channel 4", "Channel 5", "Channel 6", "Channel 7", "Channel 8", "Channel 9", "Channel 10", "Channel 11", "Channel 12", "Channel 13", "Channel 14", "Channel 15", "Channel 16"]; "Black Boxes"."Status" items=["no info", "off/false", "on/true", "Failure", "Alarm", "Status 1", "Status 2", "Status 3"]}
  in  "Version 3":T33={"Black Boxes"=[], "Calorimeters"=[], "Current Meas'"=[], "Powermeters"=[], "Cams"=[], "Img Operators"=[], "Mercury Monitors"=[], "Chillers"=[], "Triggers"=[], "Vac Controls"=[], "PP PUs"=[], "BNC555s"=[], "SRDG535s"=[], "Sequencer Data"={"Instance"="", "Snapshot: Date"="N/A", "Snapshot: Time"="N/A", "Shot Comment"=""}, "Backreflection Meas"=[]} {"Backreflection Meas"."Waveform Data"."Initial X" format="%.2e"; "SRDG535s"."Trigger Settings"."Burst Period" min=4 max=32766; "SRDG535s"."Trigger Settings"."Internal/Burst Rate (Hz)" min=0.001 max=1000000.0 format="%.3f"; "SRDG535s"."Trigger Settings"."external level (V)" min=-2.56 max=2.56 format="%.2f"; "SRDG535s"."Trigger Settings"."burst count" min=2 max=32766; "SRDG535s"."Trigger Settings"."trigger" scale=0.0..4.0; "SRDG535s"."Output Settings"."CH CD"."Mode" items=["TTL", "NIM", "ECL", "VAR"]; "SRDG535s"."Output Settings"."CH CD"."Offset (V)" min=-3.0 max=4.0 format="%.2f"; "SRDG535s"."Output Settings"."CH CD"."Amplitude (V)" min=-3.0 max=4.0 format="%.2f"; "SRDG535s"."Output Settings"."CH D"."Mode" items=["TTL", "NIM", "ECL", "VAR"]; "SRDG535s"."Output Settings"."CH D"."Offset (V)" min=-3.0 max=4.0 format="%.2f"; "SRDG535s"."Output Settings"."CH D"."Amplitude (V)" min=-3.0 max=4.0 format="%.2f"; "SRDG535s"."Output Settings"."CH C"."Mode" items=["TTL", "NIM", "ECL", "VAR"]; "SRDG535s"."Output Settings"."CH C"."Offset (V)" min=-3.0 max=4.0 format="%.2f"; "SRDG535s"."Output Settings"."CH C"."Amplitude (V)" min=-3.0 max=4.0 format="%.2f"; "SRDG535s"."Output Settings"."CH AB"."Mode" items=["TTL", "NIM", "ECL", "VAR"]; "SRDG535s"."Output Settings"."CH AB"."Offset (V)" min=-3.0 max=4.0 format="%.2f"; "SRDG535s"."Output Settings"."CH AB"."Amplitude (V)" min=-3.0 max=4.0 format="%.2f"; "SRDG535s"."Output Settings"."CH B"."Mode" items=["TTL", "NIM", "ECL", "VAR"]; "SRDG535s"."Output Settings"."CH B"."Offset (V)" min=-3.0 max=4.0 format="%.2f"; "SRDG535s"."Output Settings"."CH B"."Amplitude (V)" min=-3.0 max=4.0 format="%.2f"; "SRDG535s"."Output Settings"."CH A"."Mode" items=["TTL", "NIM", "ECL", "VAR"]; "SRDG535s"."Output Settings"."CH A"."Offset (V)" min=-3.0 max=4.0 format="%.2f"; "SRDG535s"."Output Settings"."CH A"."Amplitude (V)" min=-3.0 max=4.0 format="%.2f"; "SRDG535s"."Output Settings"."CH T0"."Mode" items=["TTL", "NIM", "ECL", "VAR"]; "SRDG535s"."Output Settings"."CH T0"."Offset (V)" min=-3.0 max=4.0 format="%.2f"; "SRDG535s"."Output Settings"."CH T0"."Amplitude (V)" min=-3.0 max=4.0 format="%.2f"; "SRDG535s"."Delay Settings"."CH D"."Delay (s)" format="%#_13g"; "SRDG535s"."Delay Settings"."CH D"."rel to" scale=0.0..3.0; "SRDG535s"."Delay Settings"."CH C"."Delay (s)" format="%#_13g"; "SRDG535s"."Delay Settings"."CH C"."rel to" scale=0.0..3.0; "SRDG535s"."Delay Settings"."CH B"."Delay (s)" format="%#_13g"; "SRDG535s"."Delay Settings"."CH B"."rel to" scale=0.0..3.0; "SRDG535s"."Delay Settings"."CH A"."Delay (s)" format="%#_13g"; "SRDG535s"."Delay Settings"."CH A"."rel to" scale=0.0..3.0; "BNC555s"."BNC555 ConfigData"."Configuration"."System"."To Gate Polarity" items=["Low", "High"]; "BNC555s"."BNC555 ConfigData"."Configuration"."System"."To Trigger Edge" items=["Rising", "Falling"]; "BNC555s"."BNC555 ConfigData"."Configuration"."System"."To Trigger Threshold" min=0.2 max=12 step=0.01 format="%.2f"; "BNC555s"."BNC555 ConfigData"."Configuration"."System"."To DCycle Off Count" min=1 max=50000 step=1; "BNC555s"."BNC555 ConfigData"."Configuration"."System"."To DCycle On Count" min=1 max=50000 step=1; "BNC555s"."BNC555 ConfigData"."Configuration"."System"."To Burst Count" min=1 max=50000 step=1; "BNC555s"."BNC555 ConfigData"."Configuration"."System"."To Trigger Mode" items=["Disabled", "Trigger", "Gate"]; "BNC555s"."BNC555 ConfigData"."Configuration"."System"."To Mode" items=["Normal", "Single", "Burst", "DCycle"]; "BNC555s"."BNC555 ConfigData"."Configuration"."System"."To Period" min=1e-06 max=20.0 step=1e-07 format="%.7f"; "BNC555s"."BNC555 ConfigData"."Configuration"."System"."To State" items=["Disabled", "Enable"]; "BNC555s"."BNC555 ConfigData"."Channel Array"."Channel Setup"."Ch Divide By Count" min=1 max=50000 step=1; "BNC555s"."BNC555 ConfigData"."Channel Array"."Channel Setup"."Ch Burst Count" min=1 max=50000 step=1; "BNC555s"."BNC555 ConfigData"."Channel Array"."Channel Setup"."Ch Mode" items=["Normal", "Single", "Burst", "Divide by"]; "BNC555s"."BNC555 ConfigData"."Channel Array"."Channel Setup"."Ch Gate" items=["Disabled", "Enabled"]; "BNC555s"."BNC555 ConfigData"."Channel Array"."Channel Setup"."Ch Gate Polarity" items=["Normal", "Complement"]; "BNC555s"."BNC555 ConfigData"."Channel Array"."Channel Setup"."Ch Polarity" items=["Normal", "Complement"]; "BNC555s"."BNC555 ConfigData"."Channel Array"."Channel Setup"."Ch Amplitude" min=1.99 max=12 step=0.01 format="%.2f"; "BNC555s"."BNC555 ConfigData"."Channel Array"."Channel Setup"."Ch Output" items=["TTL", "Adjustable"]; "BNC555s"."BNC555 ConfigData"."Channel Array"."Channel Setup"."Ch Delay" min=0.0 max=20.0 step=1e-09 format="%.9f"; "BNC555s"."BNC555 ConfigData"."Channel Array"."Channel Setup"."Ch Width" min=4e-09 max=20.0 step=1e-09 format="%.9f"; "BNC555s"."BNC555 ConfigData"."Channel Array"."Channel Setup"."Ch State" items=["Disabled", "Enable"]; "PP PUs"."State" items=["no info", "off/false/out", "on/true/in", "Failure", "Alarm", "Status 1", "Status 2", "Status 3"]; "Chillers"."State Niveau" items=["no info", "off/false", "on/true", "Failure", "Alarm"]; "Chillers"."State Temperature" items=["no info", "off/false", "on/true", "Failure", "Alarm"]; "Chillers"."State Conductivity" items=["no info", "off/false", "on/true", "Failure", "Alarm"]; "Chillers"."State Flow" items=["no info", "off/false", "on/true", "Failure", "Alarm"]; "Mercury Monitors"."Concentration [mg/m³]" format="%#_9g"; "Mercury Monitors"."State Alarm" items=["no info", "off/false", "on/true", "Failure", "Alarm"]; "Mercury Monitors"."State On/Off" items=["no info", "off/false", "on/true", "Failure", "Alarm"]; "Img Operators"."Energy"."State" items=["no info", "off/false", "on/true", "Failure", "Alarm"]; "Img Operators"."Cam Settings"."Serial Number" format="%#_12g"; "Img Operators"."Calibration"."Calibration data - Version 1"."Cam Settings"."Serial Number" format="%#_12g"; "Img Operators"."Calibration"."Status" items=["no info", "off/false", "on/true", "Failure", "Alarm"]; "Cams"."Cam Settings"."Serial Number" format="%#_12g"; "Powermeters"."Device State" items=["no info", "off/false", "on/true", "Failure", "Alarm"]; "Calorimeters"."PH Calorimeter Device Config"."Channel Gain" items=["Range: +/- 10 V", "Range: +/- 2.5 V ", "Range: +/- 1 V", "Range: +/- 0.25 V", "Range: +/- 0.1 V", "Range: +/- 0.025 V"]; "Calorimeters"."PH Calorimeter Device Config"."Channel" items=["Channel 1", "Channel 2", "Channel 3", "Channel 4", "Channel 5", "Channel 6", "Channel 7", "Channel 8", "Channel 9", "Channel 10", "Channel 11", "Channel 12", "Channel 13", "Channel 14", "Channel 15", "Channel 16"]; "Black Boxes"."Status" items=["no info", "off/false", "on/true", "Failure", "Alarm", "Status 1", "Status 2", "Status 3"]}
  in  "Version 2":T32={"Black Boxes"=[], "Calorimeters"=[], "Current Meas'"=[], "Powermeters"=[], "Cams"=[], "Img Operators"=[], "Mercury Monitors"=[], "Chillers"=[], "Triggers"=[], "Vac Controls"=[], "PP PUs"=[], "BNC555s"=[], "SRDG535s"=[], "Sequencer Data"={"Instance"="", "Snapshot: Date"="N/A", "Snapshot: Time"="N/A", "Shot Comment"=""}} {"SRDG535s"."Trigger Settings"."Burst Period" min=4 max=32766; "SRDG535s"."Trigger Settings"."Internal/Burst Rate (Hz)" min=0.001 max=1000000.0 format="%.3f"; "SRDG535s"."Trigger Settings"."external level (V)" min=-2.56 max=2.56 format="%.2f"; "SRDG535s"."Trigger Settings"."burst count" min=2 max=32766; "SRDG535s"."Trigger Settings"."trigger" scale=0.0..4.0; "SRDG535s"."Output Settings"."CH CD"."Mode" items=["TTL", "NIM", "ECL", "VAR"]; "SRDG535s"."Output Settings"."CH CD"."Offset (V)" min=-3.0 max=4.0 format="%.2f"; "SRDG535s"."Output Settings"."CH CD"."Amplitude (V)" min=-3.0 max=4.0 format="%.2f"; "SRDG535s"."Output Settings"."CH D"."Mode" items=["TTL", "NIM", "ECL", "VAR"]; "SRDG535s"."Output Settings"."CH D"."Offset (V)" min=-3.0 max=4.0 format="%.2f"; "SRDG535s"."Output Settings"."CH D"."Amplitude (V)" min=-3.0 max=4.0 format="%.2f"; "SRDG535s"."Output Settings"."CH C"."Mode" items=["TTL", "NIM", "ECL", "VAR"]; "SRDG535s"."Output Settings"."CH C"."Offset (V)" min=-3.0 max=4.0 format="%.2f"; "SRDG535s"."Output Settings"."CH C"."Amplitude (V)" min=-3.0 max=4.0 format="%.2f"; "SRDG535s"."Output Settings"."CH AB"."Mode" items=["TTL", "NIM", "ECL", "VAR"]; "SRDG535s"."Output Settings"."CH AB"."Offset (V)" min=-3.0 max=4.0 format="%.2f"; "SRDG535s"."Output Settings"."CH AB"."Amplitude (V)" min=-3.0 max=4.0 format="%.2f"; "SRDG535s"."Output Settings"."CH B"."Mode" items=["TTL", "NIM", "ECL", "VAR"]; "SRDG535s"."Output Settings"."CH B"."Offset (V)" min=-3.0 max=4.0 format="%.2f"; "SRDG535s"."Output Settings"."CH B"."Amplitude (V)" min=-3.0 max=4.0 format="%.2f"; "SRDG535s"."Output Settings"."CH A"."Mode" items=["TTL", "NIM", "ECL", "VAR"]; "SRDG535s"."Output Settings"."CH A"."Offset (V)" min=-3.0 max=4.0 format="%.2f"; "SRDG535s"."Output Settings"."CH A"."Amplitude (V)" min=-3.0 max=4.0 format="%.2f"; "SRDG535s"."Output Settings"."CH T0"."Mode" items=["TTL", "NIM", "ECL", "VAR"]; "SRDG535s"."Output Settings"."CH T0"."Offset (V)" min=-3.0 max=4.0 format="%.2f"; "SRDG535s"."Output Settings"."CH T0"."Amplitude (V)" min=-3.0 max=4.0 format="%.2f"; "SRDG535s"."Delay Settings"."CH D"."Delay (s)" format="%#_13g"; "SRDG535s"."Delay Settings"."CH D"."rel to" scale=0.0..3.0; "SRDG535s"."Delay Settings"."CH C"."Delay (s)" format="%#_13g"; "SRDG535s"."Delay Settings"."CH C"."rel to" scale=0.0..3.0; "SRDG535s"."Delay Settings"."CH B"."Delay (s)" format="%#_13g"; "SRDG535s"."Delay Settings"."CH B"."rel to" scale=0.0..3.0; "SRDG535s"."Delay Settings"."CH A"."Delay (s)" format="%#_13g"; "SRDG535s"."Delay Settings"."CH A"."rel to" scale=0.0..3.0; "BNC555s"."BNC555 ConfigData"."Configuration"."System"."To Gate Polarity" items=["Low", "High"]; "BNC555s"."BNC555 ConfigData"."Configuration"."System"."To Trigger Edge" items=["Rising", "Falling"]; "BNC555s"."BNC555 ConfigData"."Configuration"."System"."To Trigger Threshold" min=0.2 max=12 step=0.01 format="%.2f"; "BNC555s"."BNC555 ConfigData"."Configuration"."System"."To DCycle Off Count" min=1 max=50000 step=1; "BNC555s"."BNC555 ConfigData"."Configuration"."System"."To DCycle On Count" min=1 max=50000 step=1; "BNC555s"."BNC555 ConfigData"."Configuration"."System"."To Burst Count" min=1 max=50000 step=1; "BNC555s"."BNC555 ConfigData"."Configuration"."System"."To Trigger Mode" items=["Disabled", "Trigger", "Gate"]; "BNC555s"."BNC555 ConfigData"."Configuration"."System"."To Mode" items=["Normal", "Single", "Burst", "DCycle"]; "BNC555s"."BNC555 ConfigData"."Configuration"."System"."To Period" min=1e-06 max=20.0 step=1e-07 format="%.7f"; "BNC555s"."BNC555 ConfigData"."Configuration"."System"."To State" items=["Disabled", "Enable"]; "BNC555s"."BNC555 ConfigData"."Channel Array"."Channel Setup"."Ch Divide By Count" min=1 max=50000 step=1; "BNC555s"."BNC555 ConfigData"."Channel Array"."Channel Setup"."Ch Burst Count" min=1 max=50000 step=1; "BNC555s"."BNC555 ConfigData"."Channel Array"."Channel Setup"."Ch Mode" items=["Normal", "Single", "Burst", "Divide by"]; "BNC555s"."BNC555 ConfigData"."Channel Array"."Channel Setup"."Ch Gate" items=["Disabled", "Enabled"]; "BNC555s"."BNC555 ConfigData"."Channel Array"."Channel Setup"."Ch Gate Polarity" items=["Normal", "Complement"]; "BNC555s"."BNC555 ConfigData"."Channel Array"."Channel Setup"."Ch Polarity" items=["Normal", "Complement"]; "BNC555s"."BNC555 ConfigData"."Channel Array"."Channel Setup"."Ch Amplitude" min=1.99 max=12 step=0.01 format="%.2f"; "BNC555s"."BNC555 ConfigData"."Channel Array"."Channel Setup"."Ch Output" items=["TTL", "Adjustable"]; "BNC555s"."BNC555 ConfigData"."Channel Array"."Channel Setup"."Ch Delay" min=0.0 max=20.0 step=1e-09 format="%.9f"; "BNC555s"."BNC555 ConfigData"."Channel Array"."Channel Setup"."Ch Width" min=4e-09 max=20.0 step=1e-09 format="%.9f"; "BNC555s"."BNC555 ConfigData"."Channel Array"."Channel Setup"."Ch State" items=["Disabled", "Enable"]; "PP PUs"."State" items=["no info", "off/false/out", "on/true/in", "Failure", "Alarm", "Status 1", "Status 2", "Status 3"]; "Chillers"."State Niveau" items=["no info", "off/false", "on/true", "Failure", "Alarm"]; "Chillers"."State Temperature" items=["no info", "off/false", "on/true", "Failure", "Alarm"]; "Chillers"."State Conductivity" items=["no info", "off/false", "on/true", "Failure", "Alarm"]; "Chillers"."State Flow" items=["no info", "off/false", "on/true", "Failure", "Alarm"]; "Mercury Monitors"."Concentration [mg/m³]" format="%#_9g"; "Mercury Monitors"."State Alarm" items=["no info", "off/false", "on/true", "Failure", "Alarm"]; "Mercury Monitors"."State On/Off" items=["no info", "off/false", "on/true", "Failure", "Alarm"]; "Img Operators"."Energy"."State" items=["no info", "off/false", "on/true", "Failure", "Alarm"]; "Img Operators"."Cam Settings"."Serial Number" format="%#_12g"; "Img Operators"."Calibration"."Calibration data - Version 1"."Cam Settings"."Serial Number" format="%#_12g"; "Img Operators"."Calibration"."Status" items=["no info", "off/false", "on/true", "Failure", "Alarm"]; "Cams"."Cam Settings"."Serial Number" format="%#_12g"; "Powermeters"."Device State" items=["no info", "off/false", "on/true", "Failure", "Alarm"]; "Calorimeters"."PH Calorimeter Device Config"."Channel Gain" items=["Range: +/- 10 V", "Range: +/- 2.5 V ", "Range: +/- 1 V", "Range: +/- 0.25 V", "Range: +/- 0.1 V", "Range: +/- 0.025 V"]; "Calorimeters"."PH Calorimeter Device Config"."Channel" items=["Channel 1", "Channel 2", "Channel 3", "Channel 4", "Channel 5", "Channel 6", "Channel 7", "Channel 8", "Channel 9", "Channel 10", "Channel 11", "Channel 12", "Channel 13", "Channel 14", "Channel 15", "Channel 16"]; "Black Boxes"."Status" items=["no info", "off/false", "on/true", "Failure", "Alarm", "Status 1", "Status 2", "Status 3"]}
  in  "Version 1":T31 {"BNC555s"."BNC555 ConfigData"."Configuration"."System"."To Gate Polarity" items=["Low", "High"]; "BNC555s"."BNC555 ConfigData"."Configuration"."System"."To Trigger Edge" items=["Rising", "Falling"]; "BNC555s"."BNC555 ConfigData"."Configuration"."System"."To Trigger Threshold" min=0.2 max=12 step=0.01 format="%.2f"; "BNC555s"."BNC555 ConfigData"."Configuration"."System"."To DCycle Off Count" min=1 max=50000 step=1; "BNC555s"."BNC555 ConfigData"."Configuration"."System"."To DCycle On Count" min=1 max=50000 step=1; "BNC555s"."BNC555 ConfigData"."Configuration"."System"."To Burst Count" min=1 max=50000 step=1; "BNC555s"."BNC555 ConfigData"."Configuration"."System"."To Trigger Mode" items=["Disabled", "Trigger", "Gate"]; "BNC555s"."BNC555 ConfigData"."Configuration"."System"."To Mode" items=["Normal", "Single", "Burst", "DCycle"]; "BNC555s"."BNC555 ConfigData"."Configuration"."System"."To Period" min=1e-06 max=20.0 step=1e-07 format="%.7f"; "BNC555s"."BNC555 ConfigData"."Configuration"."System"."To State" items=["Disabled", "Enable"]; "BNC555s"."BNC555 ConfigData"."Channel Array"."Channel Setup"."Ch Divide By Count" min=1 max=50000 step=1; "BNC555s"."BNC555 ConfigData"."Channel Array"."Channel Setup"."Ch Burst Count" min=1 max=50000 step=1; "BNC555s"."BNC555 ConfigData"."Channel Array"."Channel Setup"."Ch Mode" items=["Normal", "Single", "Burst", "Divide by"]; "BNC555s"."BNC555 ConfigData"."Channel Array"."Channel Setup"."Ch Gate" items=["Disabled", "Enabled"]; "BNC555s"."BNC555 ConfigData"."Channel Array"."Channel Setup"."Ch Gate Polarity" items=["Normal", "Complement"]; "BNC555s"."BNC555 ConfigData"."Channel Array"."Channel Setup"."Ch Polarity" items=["Normal", "Complement"]; "BNC555s"."BNC555 ConfigData"."Channel Array"."Channel Setup"."Ch Amplitude" min=1.99 max=12 step=0.01 format="%.2f"; "BNC555s"."BNC555 ConfigData"."Channel Array"."Channel Setup"."Ch Output" items=["TTL", "Adjustable"]; "BNC555s"."BNC555 ConfigData"."Channel Array"."Channel Setup"."Ch Delay" min=0.0 max=20.0 step=1e-09 format="%.9f"; "BNC555s"."BNC555 ConfigData"."Channel Array"."Channel Setup"."Ch Width" min=4e-09 max=20.0 step=1e-09 format="%.9f"; "BNC555s"."BNC555 ConfigData"."Channel Array"."Channel Setup"."Ch State" items=["Disabled", "Enable"]; "PP PUs"."State" items=["no info", "off/false/out", "on/true/in", "Failure", "Alarm", "Status 1", "Status 2", "Status 3"]; "Chillers"."State Niveau" items=["no info", "off/false", "on/true", "Failure", "Alarm"]; "Chillers"."State Temperature" items=["no info", "off/false", "on/true", "Failure", "Alarm"]; "Chillers"."State Conductivity" items=["no info", "off/false", "on/true", "Failure", "Alarm"]; "Chillers"."State Flow" items=["no info", "off/false", "on/true", "Failure", "Alarm"]; "Mercury Monitors"."Concentration [mg/m³]" format="%#_9g"; "Mercury Monitors"."State Alarm" items=["no info", "off/false", "on/true", "Failure", "Alarm"]; "Mercury Monitors"."State On/Off" items=["no info", "off/false", "on/true", "Failure", "Alarm"]; "Img Operators"."Energy"."State" items=["no info", "off/false", "on/true", "Failure", "Alarm"]; "Img Operators"."Cam Settings"."Serial Number" format="%#_12g"; "Img Operators"."Calibration"."Calibration data - Version 1"."Cam Settings"."Serial Number" format="%#_12g"; "Img Operators"."Calibration"."Status" items=["no info", "off/false", "on/true", "Failure", "Alarm"]; "Cams"."Cam Settings"."Serial Number" format="%#_12g"; "Powermeters"."Device State" items=["no info", "off/false", "on/true", "Failure", "Alarm"]; "Calorimeters"."PH Calorimeter Device Config"."Channel Gain" items=["Range: +/- 10 V", "Range: +/- 2.5 V ", "Range: +/- 1 V", "Range: +/- 0.25 V", "Range: +/- 0.1 V", "Range: +/- 0.025 V"]; "Calorimeters"."PH Calorimeter Device Config"."Channel" items=["Channel 1", "Channel 2", "Channel 3", "Channel 4", "Channel 5", "Channel 6", "Channel 7", "Channel 8", "Channel 9", "Channel 10", "Channel 11", "Channel 12", "Channel 13", "Channel 14", "Channel 15", "Channel 16"]; "Black Boxes"."Status" items=["no info", "off/false", "on/true", "Failure", "Alarm", "Status 1", "Status 2", "Status 3"]}
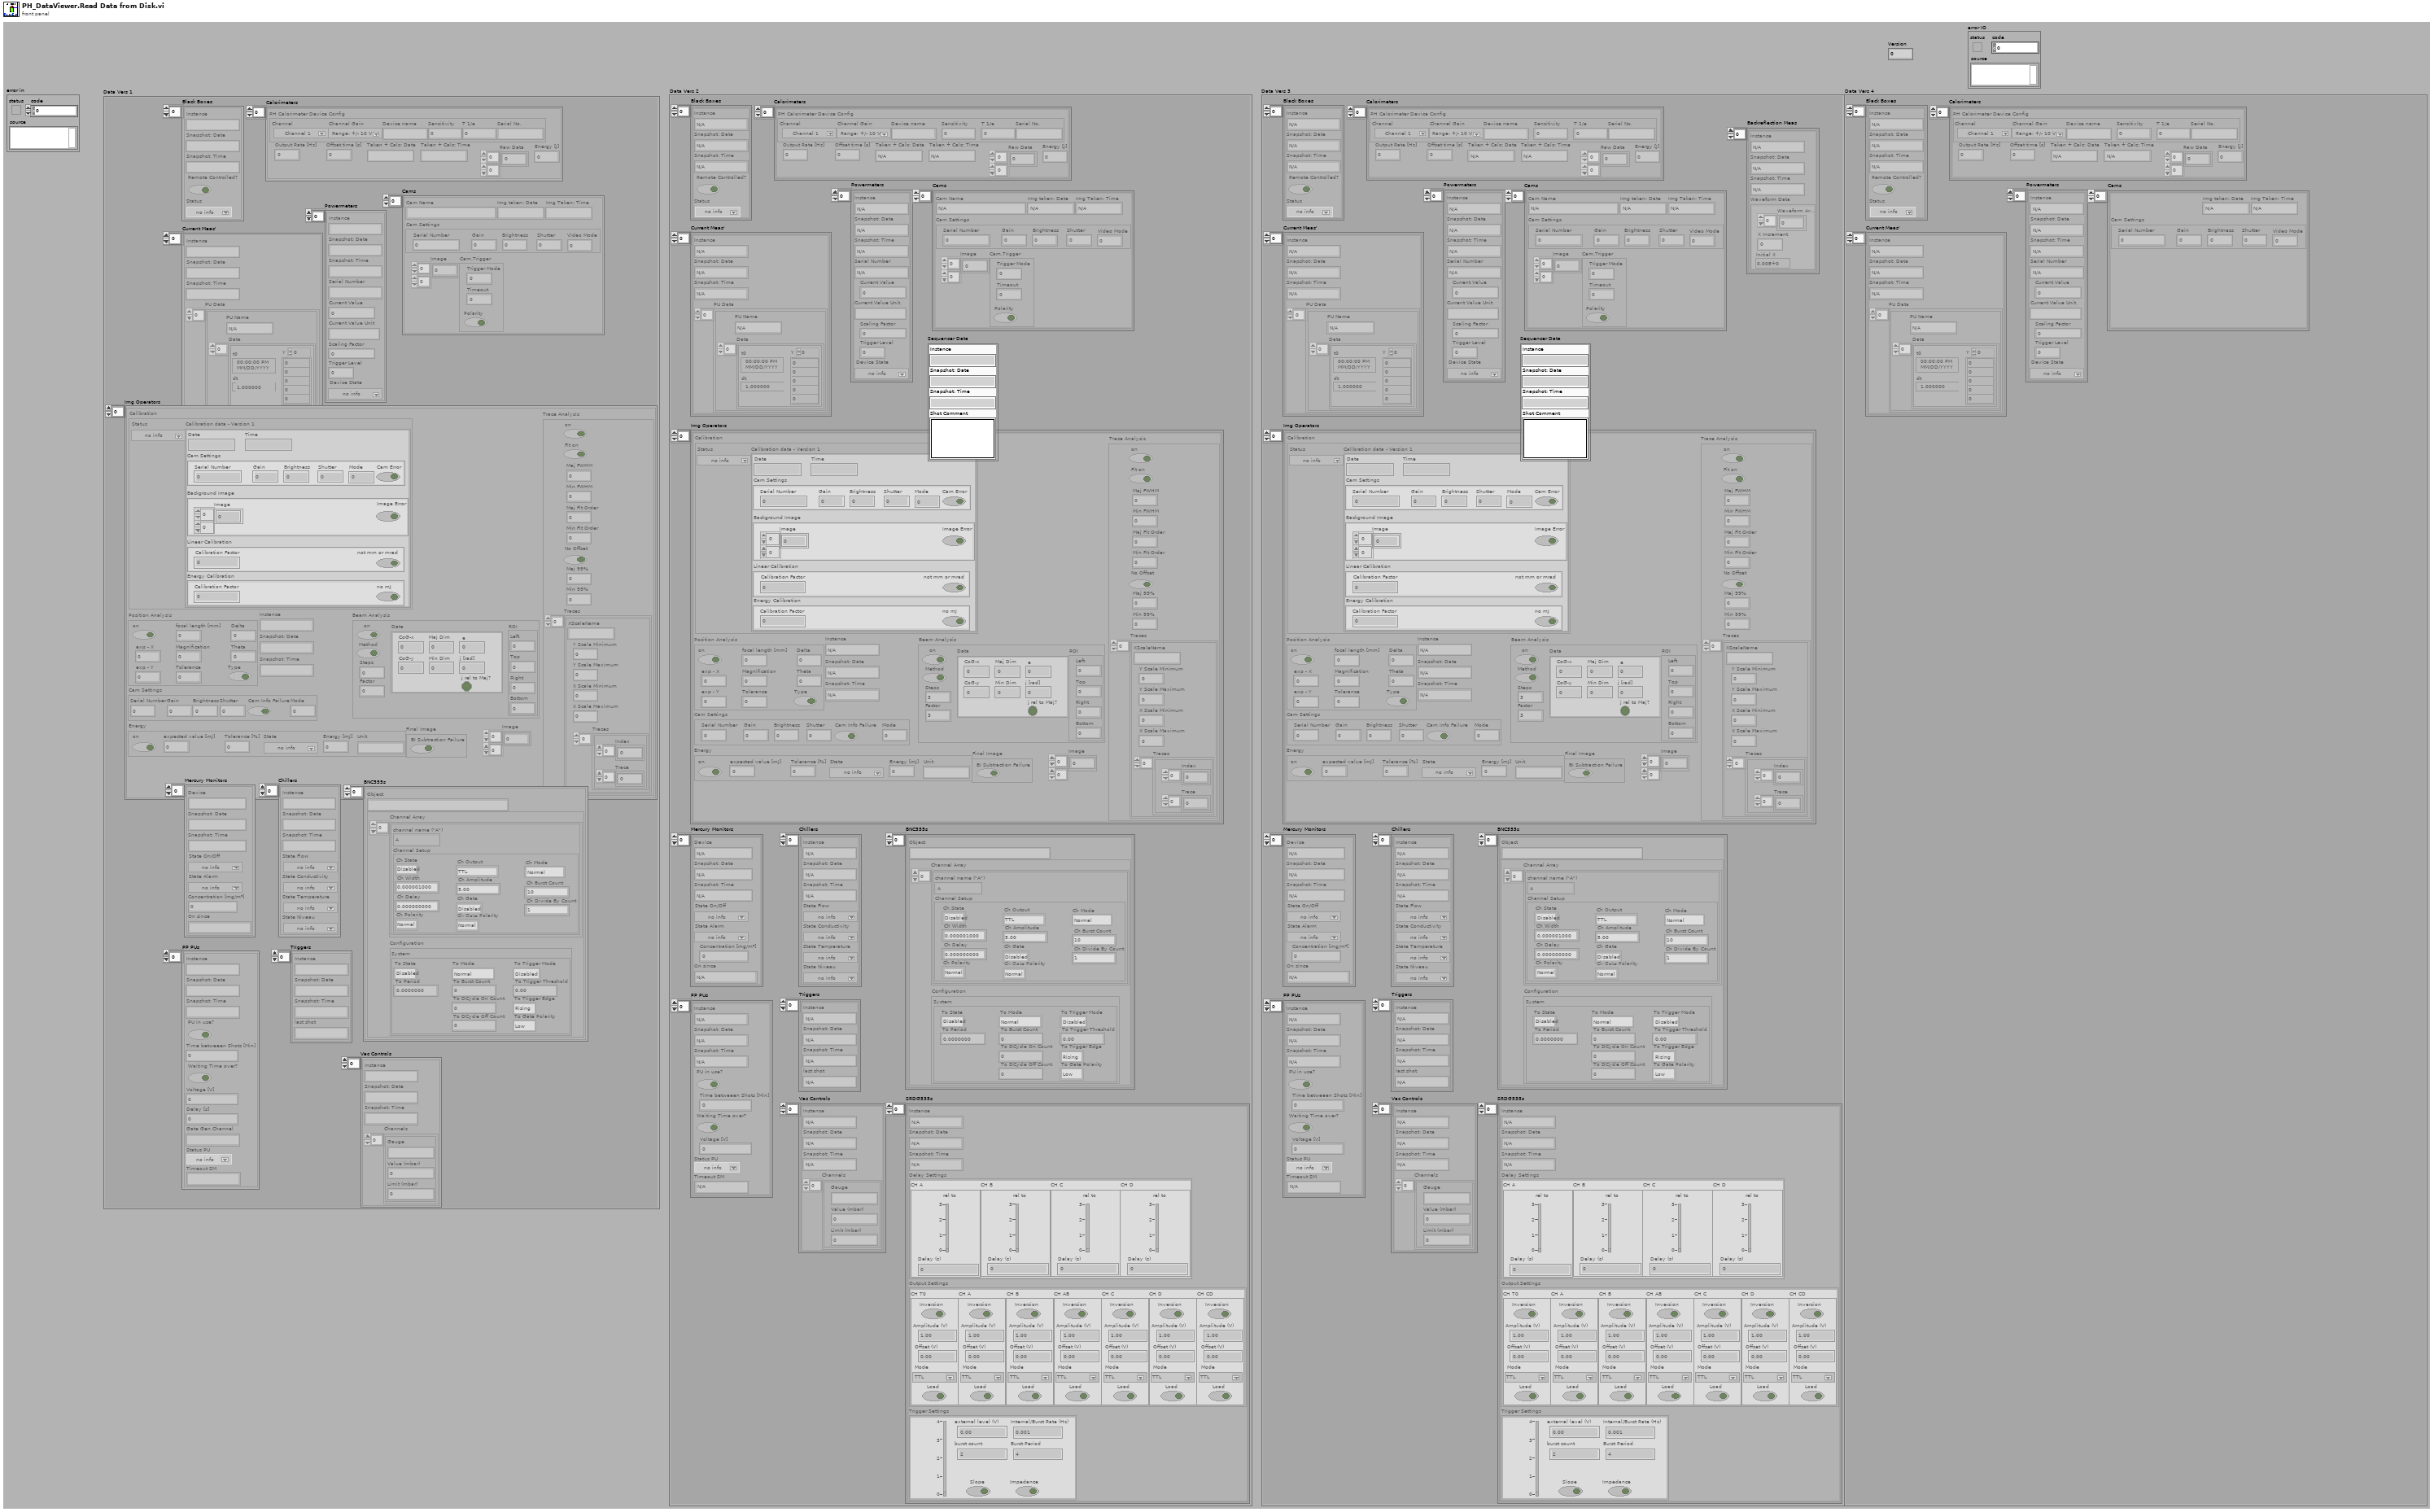
[diagram p1: front panel]
types:
  T1 = typedef "PH_DataViewer.lvlib/PHELIX_Data_Vers4.ctl" = cluster{"Black Boxes":T2[], "Calorimeters":T3[], "Current Meas'":T7[], "Powermeters":T8[], "Cams":T10[], "Img Operators":T12[], "Mercury Monitors":T15[], "Chillers":T16[], "Triggers":T17[], "Vac Controls":T18[], "PP PUs":T19[], "BNC555s":cluster{"Object":string, "BNC555 ConfigData":T21}[], "SRDG535s":T22[], "Sequencer Data":T27, "Backreflection Meas":T28[], "OO Spectrometer":T29[]}
  T2 = typedef "PH_DataViewer.lvlib/PH_Blackbox.Data.ctl" = cluster{"Instance":string, "Snapshot: Date":string, "Snapshot: Time":string, "Remote Controlled?":bool, "Status":i32}
  T3 = typedef "PH_DataViewer.lvlib/PH_Calorimater_USB.Data.ctl" = cluster{"PH Calorimeter Device Config":T4, "Output Rate [Hz]":i32, "Offset time [s]":dbl, "Taken + Calc: Date":string, "Taken + Calc: Time":string, "Raw Data":dbl[][], "Energy [J]":dbl}
  T4 = typedef "PH_Calorimeter_USB.lvlib/PH_Calorimeter_USB.Device Config.ctl" = cluster{"Channel":T5, "Channel Gain":T6, "Device name":string, "Sensitivity":dbl, "T 1/e":dbl, "Serial No.":string}
  T5 = typedef "PH_Calorimeter_USB.lvlib/PH_Calorimeter_USB.Channel.ctl" = u16
  T6 = typedef "PH_Calorimeter_USB.lvlib/PH_Calorimeter_USB.Channel Gain.ctl" = u16
  T7 = typedef "PH_DataViewer.lvlib/PH_CurrentMeas.Data.ctl" = cluster{"Instance":string, "Snapshot: Date":string, "Snapshot: Time":string, "PU Data":cluster{"Data":waveform(dbl)[], "PU Name":string}[]}
  T8 = typedef "PH_DataViewer.lvlib/PH_gentec_Powermeter.Data.ctl" = cluster{"Instance":string, "Snapshot: Date":string, "Snapshot: Time":string, "Serial Number":string, "Current Value":dbl, "Current Value Unit":string, "Scaling Factor":dbl, "Trigger Level":dbl, "Device State":T9}
  T9 = typedef "PH_DataViewer.lvlib/PH_DataViewer.Device State.ctl" = i32
  T10 = typedef "PH_DataViewer.lvlib/PH_IEEE1394Camera.Data.ctl" = cluster{"Cam Name":string, "Img taken: Date":string, "Img Taken: Time":string, "Cam Settings":T11, "Image":sgl[][], "Cam.Trigger":cluster{"Trigger Mode":u16, "Timeout":u32, "Polarity":bool}}
  T11 = typedef "PH_DataViewer.lvlib/PH_IEEE1394Camera.Settings.ctl" = cluster{"Serial Number":dbl, "Gain":i32, "Brightness":i32, "Shutter":i32, "Video Mode":i32}
  T12 = typedef "PH_DataViewer.lvlib/PH_ImageOperator.Data.ctl" = cluster{"Instance":string, "Snapshot: Date":string, "Snapshot: Time":string, "Calibration":cluster{"Status":T9, "Calibration data - Version 1":T13}, "Position Analysis":cluster{"on":bool, "exp - X":i32, "exp - Y":i32, "focal length [mm]":dbl, "Magnification":dbl, "Delta":dbl, "Theta":dbl, "Tolerance":dbl, "Type":bool}, "Beam Analysis":cluster{"on":bool, "Data":T14, "Method":bool, "Steps":i32, "Factor":i32, "ROI":cluster{"Left":i32, "Top":i32, "Right":i32, "Bottom":i32}}, "Cam Settings":cluster{"Serial Number":dbl, "Gain":i32, "Brightness":i32, "Shutter":i32, "Cam Info Failure":bool, "Mode":i32}, "Energy":cluster{"on":bool, "expected value [mJ]":dbl, "Tolerance [%]":dbl, "State":T9, "Energy [mJ]":dbl, "Unit":string}, "Image":dbl[][], "Final Image":cluster{"BI Subtraction Failure":bool}, "Trace Analysis":cluster{"on":bool, "Fit on":bool, "Maj FWHM":dbl, "Min FWHM":dbl, "Maj Fit Order":i32, "Min Fit Order":i32, "No Offset":bool, "Maj 99%":dbl, "Min 99%":dbl, "Traces":cluster{"XScaleName":string, "Y Scale Minimum":sgl, "Y Scale Maximum":sgl, "X Scale Minimum":sgl, "X Scale Maximum":sgl, "Traces":cluster{"Index":sgl[], "Trace":dbl[]}[]}[]}}
  T13 = typedef "PH_ImageCalibrator.lvlib/PH_ImageCalibrator.Calibration Data - Version 1.ctl" = cluster{"Date":string, "Time":string, "Cam Settings":cluster{"Serial Number":dbl, "Gain":i32, "Brightness":i32, "Shutter":i32, "Cam Error":bool, "Mode":i32}, "Background Image":cluster{"Image":dbl[][], "Image Error":bool}, "Linear Calibration":cluster{"Calibration Factor":dbl, "not mm or mrad":bool}, "Energy Calibration":cluster{"Calibration Factor":dbl, "no mJ":bool}}
  T14 = typedef "PH_ImageOperator.lvlib/PH_ImageOperator.Beam Analysis Data.ctl" = cluster{"CoG-x":sgl, "CoG-y":sgl, "Maj Dim":dbl, "Min Dim":dbl, "Ellipticity":dbl, "Azimuth Angle [rad]":dbl, "Azi Angle rel to Maj?":bool}
  T15 = typedef "PH_DataViewer.lvlib/PH_Mercury_Monitor.Data.ctl" = cluster{"Device":string, "Snapshot: Date":string, "Snapshot: Time":string, "State On/Off":T9, "State Alarm":T9, "Concentration [mg/m³]":dbl, "On since":string}
  T16 = typedef "PH_DataViewer.lvlib/PH_PA_Chiller.Data.ctl" = cluster{"Instance":string, "Snapshot: Date":string, "Snapshot: Time":string, "State Flow":T9, "State Conductivity":T9, "State Temperature":T9, "State Niveau":T9}
  T17 = typedef "PH_DataViewer.lvlib/PH_PP_Trigger.Data.ctl" = cluster{"Instance":string, "Snapshot: Date":string, "Snapshot: Time":string, "last shot":string}
  T18 = typedef "PH_DataViewer.lvlib/PH_VacuumControl.Data.ctl" = cluster{"Instance":string, "Snapshot: Date":string, "Snapshot: Time":string, "Channels":cluster{"Gauge":string, "Value (mbar)":dbl, "Limit (mbar)":dbl}[]}
  T19 = typedef "PH_DataViewer.lvlib/PH_Common.PP PU Data Vers2.ctl" = cluster{"Instance":string, "Snapshot: Date":string, "Snapshot: Time":string, "PU in use?":bool, "Time betweeen Shots [Min]":dbl, "Waiting Time over?":bool, "Voltage [V]":dbl, "State":T20, "Timeout SM":string}
  T20 = typedef "PH_StatusHandler.lvlib/PH_StatusHandler.Status.ctl" = i16
  T21 = typedef "PH_DataViewer.lvlib/BNC555.Data.ctl" = cluster{"Channel Array":cluster{"channel name (\"A\")":string, "Channel Setup":cluster{"Ch State":i8, "Ch Width":dbl, "Ch Delay":dbl, "Ch Output":i8, "Ch Amplitude":sgl, "Ch Polarity":i8, "Ch Gate Polarity":i8, "Ch Gate":i8, "Ch Mode":i8, "Ch Burst Count":i32, "Ch Divide By Count":i32}}[], "Configuration":cluster{"System":cluster{"To State":i8, "To Period":dbl, "To Mode":i8, "To Trigger Mode":i8, "To Burst Count":i32, "To DCycle On Count":i32, "To DCycle Off Count":i32, "To Trigger Threshold":sgl, "To Trigger Edge":i8, "To Gate Polarity":i8}}}
  T22 = typedef "PH_DataViewer.lvlib/SRDG535.Data.ctl" = cluster{"Instance":string, "Snapshot: Date":string, "Snapshot: Time":string, "Delay Settings":T23, "Output Settings":T24, "Trigger Settings":T26}
  T23 = typedef "SRDG535.lvlib/SRDG535.Delay.ctl" = cluster{"CH A":cluster{"rel to":u32, "Delay (s)":dbl}, "CH B":cluster{"rel to":u32, "Delay (s)":dbl}, "CH C":cluster{"rel to":u32, "Delay (s)":dbl}, "CH D":cluster{"rel to":u32, "Delay (s)":dbl}}
  T24 = typedef "SRDG535.lvlib/SRDG535.Output.ctl" = cluster{"CH T0":T25, "CH A":T25, "CH B":T25, "CH AB":T25, "CH C":T25, "CH D":T25, "CH CD":T25}
  T25 = typedef "SRDG535.lvlib/SRDG535.Channel Output.ctl" = cluster{"Inversion":bool, "Amplitude (V)":dbl, "Offset (V)":dbl, "Mode":i32, "Load":bool}
  T26 = typedef "SRDG535.lvlib/SRDG535.Trigger.ctl" = cluster{"trigger":u32, "Impedance":bool, "Slope":bool, "burst count":i32, "external level (V)":sgl, "Internal/Burst Rate (Hz)":dbl, "Burst Period":i32}
  T27 = typedef "PH_DataViewer.lvlib/PH_Sequencer.Data.ctl" = cluster{"Instance":string, "Snapshot: Date":string, "Snapshot: Time":string, "Shot Comment":string}
  T28 = typedef "PH_DataViewer.lvlib/PH_BackreflectionMeas.Data.ctl" = cluster{"Instance":string, "Snapshot: Date":string, "Snapshot: Time":string, "Waveform Data":cluster{"Waveform Array":dbl[], "X Increment":dbl, "Initial X":dbl}}
  T29 = typedef "PH_DataViewer.lvlib/PH_OceanOpticsSpectrometer.Data.ctl" = cluster{"Instance":string, "Date":string, "Time":string, "Wavelength Bins":dbl[], "Spectrum by Pixels":dbl[]}
  T30 = typedef "PH_DataViewer.lvlib/PH_Common.PP PU Data.ctl" = cluster{"Instance":string, "Snapshot: Date":string, "Snapshot: Time":string, "PU in use?":bool, "Time betweeen Shots [Min]":dbl, "Waiting Time over?":bool, "Voltage [V]":dbl, "Delay [s]":dbl, "Gate Gen Channel":string, "State":T20, "Timeout SM":string}
  T31 = cluster{"Black Boxes":T2[], "Calorimeters":T3[], "Current Meas'":T7[], "Powermeters":T8[], "Cams":T10[], "Img Operators":T12[], "Mercury Monitors":T15[], "Chillers":T16[], "Triggers":T17[], "Vac Controls":T18[], "PP PUs":T30[], "BNC555s":cluster{"Object":string, "BNC555 ConfigData":T21}[]}
  T32 = typedef "PH_DataViewer.lvlib/PHELIX_Data_Vers2.ctl" = cluster{"Black Boxes":T2[], "Calorimeters":T3[], "Current Meas'":T7[], "Powermeters":T8[], "Cams":T10[], "Img Operators":T12[], "Mercury Monitors":T15[], "Chillers":T16[], "Triggers":T17[], "Vac Controls":T18[], "PP PUs":T19[], "BNC555s":cluster{"Object":string, "BNC555 ConfigData":T21}[], "SRDG535s":T22[], "Sequencer Data":T27}
  T33 = typedef "PH_DataViewer.lvlib/PHELIX_Data_Vers3.ctl" = cluster{"Black Boxes":T2[], "Calorimeters":T3[], "Current Meas'":T7[], "Powermeters":T8[], "Cams":T10[], "Img Operators":T12[], "Mercury Monitors":T15[], "Chillers":T16[], "Triggers":T17[], "Vac Controls":T18[], "PP PUs":T19[], "BNC555s":cluster{"Object":string, "BNC555 ConfigData":T21}[], "SRDG535s":T22[], "Sequencer Data":T27, "Backreflection Meas":T28[]}
  T34 = enum16{"open", "replace", "create", "open or create", "replace or create", "replace or create with confirmation"}
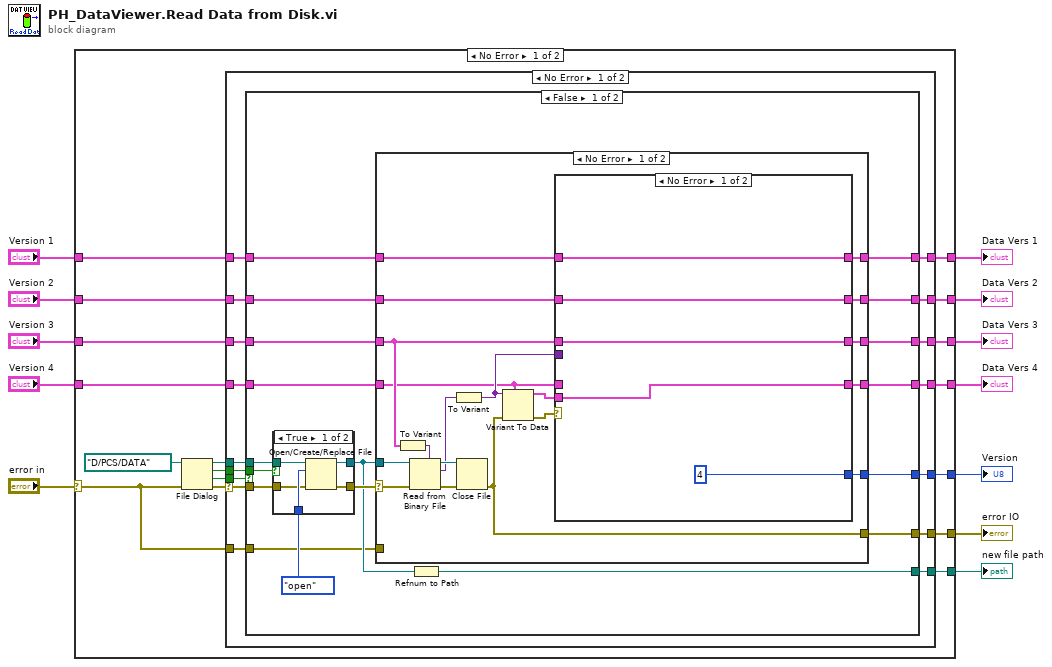
[diagram p0: block diagram]
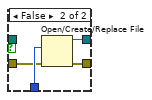
[diagram p2: hidden frame]
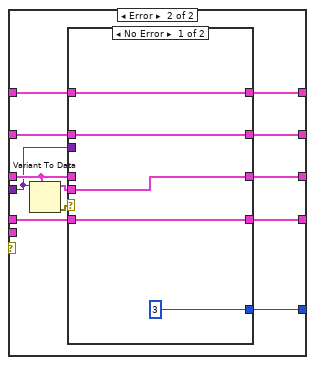
[diagram p3: hidden frame]
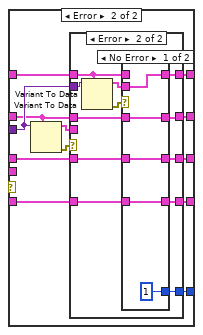
[diagram p4: hidden frame]
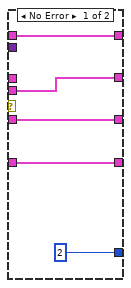
[diagram p5: hidden frame]
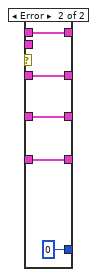
[diagram p6: hidden frame]
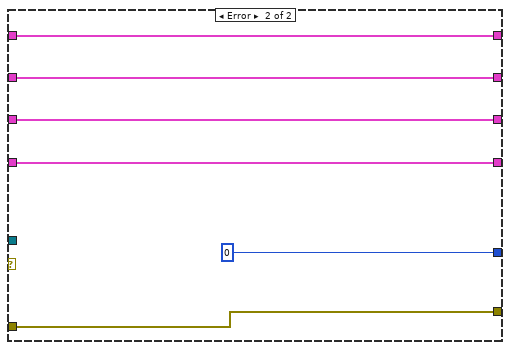
[diagram p7: hidden frame]
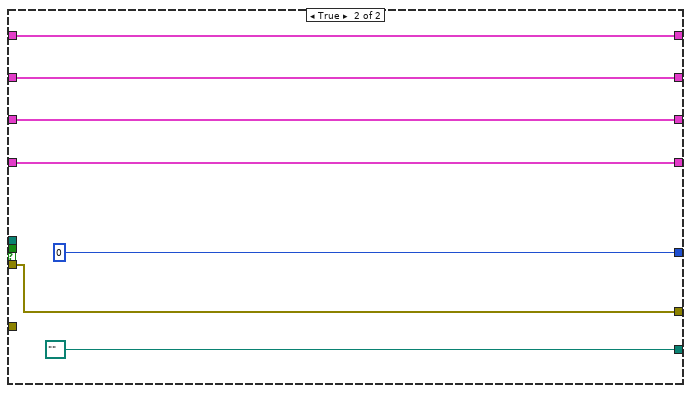
[diagram p8: hidden frame]
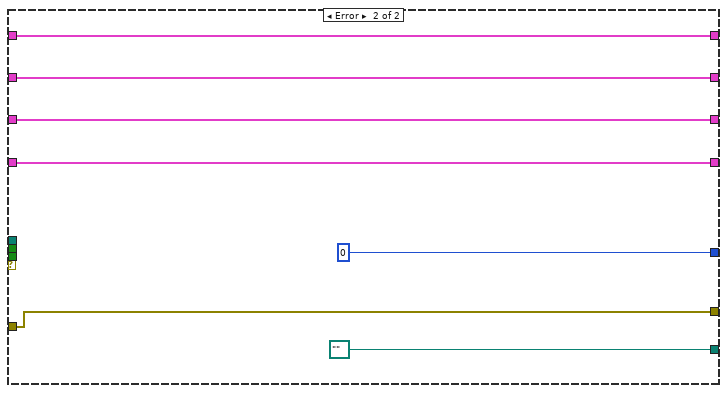
[diagram p9: hidden frame]
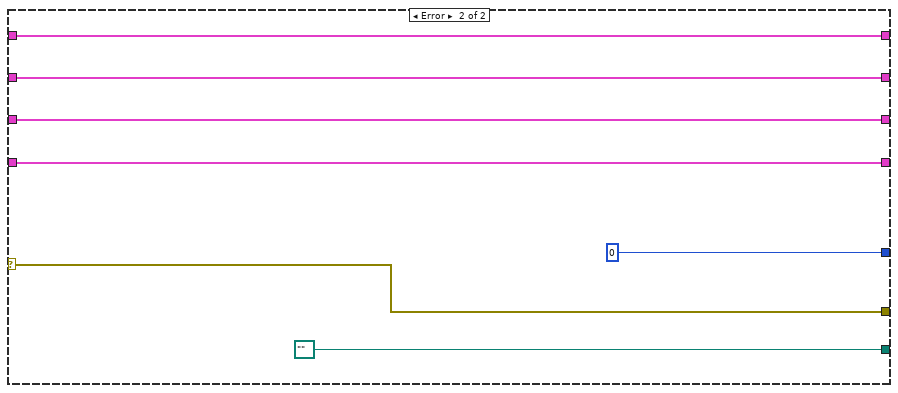
[diagram p10: hidden frame]
diagram:
  n1 = case shown="No Error" "error in" {
    selector: "error in" -> [w16 w175]
    tunnel: [w29 w179] -> w8
    tunnel: "Version 1" -> [w28 w179]
    tunnel: [w19 path "" ("new file path")] -> w1
    tunnel: [w27 u8 0 ("Version")] -> w11
    tunnel: "Version 2" -> [w26 w177]
    tunnel: [w25 w177] -> w9
    tunnel: "Version 3" -> [w24 w176]
    tunnel: [w23 w176] -> w10
    tunnel: [w22 w175] -> w12
    tunnel: "Version 4" -> [w21 w174]
    tunnel: [w20 w174] -> w2
    frame No Error {
      n2 = File Dialog(8:w16, 11:path "D:/PCS/DATA" ("start path")) -> (0:w15:errorcluster, 1:w14:bool, 2:w13:bool, 3:w17:path)  [unwired: 5 in]
      n3 = case shown="No Error" w15 {
        selector: w15 -> [w32 _]
        tunnel: [w45 w172] -> w29
        tunnel: w28 -> [w44 w172]
        tunnel: [w43 u8 0 ("Version")] -> w27
        tunnel: w26 -> [w42 w171]
        tunnel: [w41 w171] -> w25
        tunnel: w24 -> [w40 w170]
        tunnel: [w39 w170] -> w23
        tunnel: [w38 w167] -> w22
        tunnel: w21 -> [w37 w169]
        tunnel: [w36 w169] -> w20
        tunnel: [w35 path ""] -> w19
        tunnel: w17 -> [w34 _]
        tunnel: w16 -> [w33 w167]
        tunnel: w14 -> [w31 _]
        tunnel: w13 -> [w30 _]
        frame No Error {
          n4 = case shown="False" w31 {
            tunnel: [w63 w165] -> w45
            tunnel: w44 -> [w61 w165]
            tunnel: [w60 u8 0 ("Version")] -> w43
            tunnel: w42 -> [w59 w164]
            tunnel: [w58 w164] -> w41
            tunnel: w40 -> [w57 w163]
            tunnel: [w56 w163] -> w39
            tunnel: [w55 w160] -> w38
            tunnel: w37 -> [w54 w162]
            tunnel: [w53 w162] -> w36
            tunnel: [w51 path ""] -> w35
            tunnel: w34 -> [w49 _]
            tunnel: w33 -> [w48 _]
            tunnel: w32 -> [w47 w160]
            tunnel: w30 -> [w46 _]
            frame False {
              n5 = case shown="True" w46 {
                tunnel: [w68 w72] -> w62
                tunnel: T34."open" ("operation (0:open)") -> [w67 w71]
                tunnel: [w66 w70] -> w50
                tunnel: w49 -> [w65 _]
                tunnel: w47 -> [w64 w69]
                frame True {
                  n6 = Open/Create/Replace File(file path (use dialog)=w65, error in=w64, operation (0:open)=w67) -> (refnum out=w66:refnum<file>, error out=w68:errorcluster)  [unwired: 3 in, 1 out]
                }
                frame False {
                  n7 = Open/Create/Replace File(error in=w69, operation (0:open)=w71) -> (refnum out=w70:refnum<file>, error out=w72:errorcluster)  [unwired: 4 in, 1 out]
                }
              }
              n8 = case shown="No Error" w62 {
                selector: w62 -> [w88 _]
                tunnel: w50 -> [w91 _]
                tunnel: [w82 w158] -> w63
                tunnel: w61 -> [w86 w158]
                tunnel: w48 -> [_ w154]
                tunnel: [w80 u8 0 ("Version")] -> w60
                tunnel: w59 -> [w85 w156]
                tunnel: [w83 w156] -> w58
                tunnel: w57 -> [w81 w155]
                tunnel: [w84 w155] -> w56
                tunnel: [w79 w154] -> w55
                tunnel: w54 -> [w75 w153]
                tunnel: [w74 w153] -> w53
                frame No Error {
                  n9 = To Variant(anything=w81) -> (Variant=w87:variant)
                  n10 = Read from Binary File(5:w87, 8:w88, 11:w91) -> (0:w89:errorcluster, 2:w78:variant, 3:w90:refnum<file>)  [unwired: 3 in, 1 out]
                  n11 = To Variant(anything=w78) -> (Variant=w77:variant)
                  n12 = Close File(refnum=w90, error in=w89) -> (error out=w79:errorcluster)  [unwired: 1 out]
                  n13 = Variant To Data(error in=w79, type=w75, Variant=w77) -> (data=w73:T1, error out=w76:errorcluster)
                  n14 = case shown="No Error" w76 {
                    tunnel: w86 -> [w95 w108]
                    tunnel: w85 -> [w94 w107]
                    tunnel: [w93 w105] -> w84
                    tunnel: [w94 w103] -> w83
                    tunnel: [w95 w102] -> w82
                    tunnel: w81 -> [w93 w101]
                    tunnel: [u8 4 w100] -> w80
                    tunnel: w77 -> [_ w99]
                    tunnel: w75 -> [_ w98]
                    tunnel: [w96 w97] -> w74
                    tunnel: w73 -> [w96 _]
                    frame No Error {
                    }
                    frame Error {
                      n15 = Variant To Data(type=w101, Variant=w99) -> (data=w104:T33, error out=w106:errorcluster)  [unwired: 1 in]
                      n16 = case shown="No Error" w106 {
                        tunnel: w99 -> [_ w125]
                        tunnel: w108 -> [w111 w124]
                        tunnel: w107 -> [w112 w117]
                        tunnel: [w113 w119] -> w105
                        tunnel: w104 -> [w113 _]
                        tunnel: [w112 w121] -> w103
                        tunnel: [w111 w122] -> w102
                        tunnel: w101 -> [_ w118]
                        tunnel: [u8 3 w116] -> w100
                        tunnel: w98 -> [w109 w115]
                        tunnel: [w109 w114] -> w97
                        frame No Error {
                        }
                        frame Error {
                          n17 = Variant To Data(type=w117, Variant=w125) -> (data=w120:T32, error out=w123:errorcluster)  [unwired: 1 in]
                          n18 = case shown="Error" w123 {
                            tunnel: w125 -> [_ w142]
                            tunnel: w124 -> [w130 w133]
                            tunnel: [w130 w135] -> w122
                            tunnel: [w129 w136] -> w121
                            tunnel: w120 -> [w129 _]
                            tunnel: [w128 w138] -> w119
                            tunnel: w118 -> [w128 w139]
                            tunnel: w117 -> [_ w137]
                            tunnel: [u8 2 w141] -> w116
                            tunnel: w115 -> [w126 w132]
                            tunnel: [w126 w131] -> w114
                            frame No Error {
                            }
                            frame Error {
                              n19 = Variant To Data(type=w133, Variant=w142) -> (data=w134:T31, error out=w140:errorcluster)  [unwired: 1 in]
                              n20 = case shown="No Error" w140 {
                                tunnel: [u8 1 u8 0] -> w141
                                tunnel: w139 -> [w146 w150]
                                tunnel: [w146 w150] -> w138
                                tunnel: w137 -> [w145 w151]
                                tunnel: [w145 w151] -> w136
                                tunnel: [w144 w152] -> w135
                                tunnel: w134 -> [w144 _]
                                tunnel: w133 -> [_ w152]
                                tunnel: w132 -> [w143 w148]
                                tunnel: [w143 w148] -> w131
                                frame No Error {
                                }
                                frame Error {
                                }
                              }
                            }
                          }
                        }
                      }
                    }
                  }
                }
                frame Error {
                }
              }
              n21 = Refnum to Path(1:w50) -> (0:w51:path)
            }
            frame True {
            }
          }
        }
        frame Error {
        }
      }
    }
    frame Error {
    }
  }
  "error IO" <- w12
  "Version" <- w11
  "Data Vers 3" <- w10
  "Data Vers 2" <- w9
  "Data Vers 1" <- w8
  "new file path" <- w1
  "Data Vers 4" <- w2
